vi "RIB Req - UDP Init.vi"(0 "Limits File Path":path, 5 "Results File Path":path, 11 "error in":errorcluster) -> (4 "Results Data Array":string[][](array[string]), 15 "error out":errorcluster)   [LabVIEW 2024]
doc: "Template test"
uses:
  <vilib>/addons/_JKI Toolkits/State Machine/_JKI_lib_State_Machine.llb/Select State(s)_err__jki_lib_state_machine.vi
  <vilib>/DAQmx/write.llb/DAQmx Write (Digital 1D Bool 1Chan 1Samp).vi
  <vilib>/addons/_JKI Toolkits/State Machine/_JKI_lib_State_Machine.llb/Select State(s)_bool__jki_lib_state_machine.vi
  <vilib>/DAQmx/read.llb/DAQmx Read (Digital 1D Bool 1Chan 1Samp).vi
  <vilib>/addons/_JKI Toolkits/State Machine/_JKI_lib_State_Machine.llb/Periodic Trigger__ogtk__JKI-SM__jki_lib_state_machine.vi
  <userlib>/_OpenG.lib/file/file.llb/Strip Path Extension - String__ogtk.vi
  <vilib>/Utility/file.llb/Read Delimited Spreadsheet (string).vi
  <vilib>/DAQmx/create/channels.llb/DAQmx Create Channel (DO-Digital Output).vi
  <vilib>/DAQmx/miscellaneous.llb/DAQmx Fill In Error Info.vi
  <userlib>/_OpenG.lib/file/file.llb/openg_file.lvlib
  <userlib>/_OpenG.lib/appcontrol/appcontrol.llb/openg_application_control.lvlib
  <userlib>/_OpenG.lib/time/time.llb/openg_time.lvlib
  <vilib>/Utility/file.llb/Write Delimited Spreadsheet (string).vi
panel:
  out "Connect Fail":string
  out "Connect":string
  out "Timeout (Read States) 4":dbl(slide) scale=0.0..30.0
  out "Timeout (Read States) 3":dbl(slide) scale=0.0..30.0
  out "Timeout (Read States) 2":dbl(slide) scale=0.0..30.0
  out "Timeout (Read States)":dbl(slide) scale=0.0..30.0
  out "element":string
  out "5A Test":bool
  out "ROV A Enabled":bool
  out "ROV B Enabled":bool
  out "TMS Enabled":bool
  out "Wait for Start":bool
  out "Normal Operation":bool
  in  "Read Normal Operation":string
  in  "Read Wait for Start":string
  in  "Read TMS":string
  in  "Read ROV B":string
  in  "Read ROV A":string
  in  "Connect":string
  in  "Connect Fail":string
  out "Results Data 10":string[](array[string])
  out "Results Data 9":string[](array[string])
  out "Results Data 8":string[](array[string])
  out "Results Data 7":string[](array[string])
  out "Results Data 6":string[](array[string])
  out "Results Data 5":string[](array[string])
  out "Results Data 4":string[](array[string])
  in  "5A Test":bool
  out "Results Data 3":string[](array[string])
  in  "task out":refnum<k21>
  out "Timeout (5A)":dbl(slide) scale=0.0..5.0
  out "Timeout (Read UDP)":dbl(slide) scale=0.0..20.0
  out "Results Data 2":string[](array[string])
  in  "UDP Read":string
  in  "connection ID":refnum<k16>
  in  "Exit":bool
  # "UDP Initialise Test"
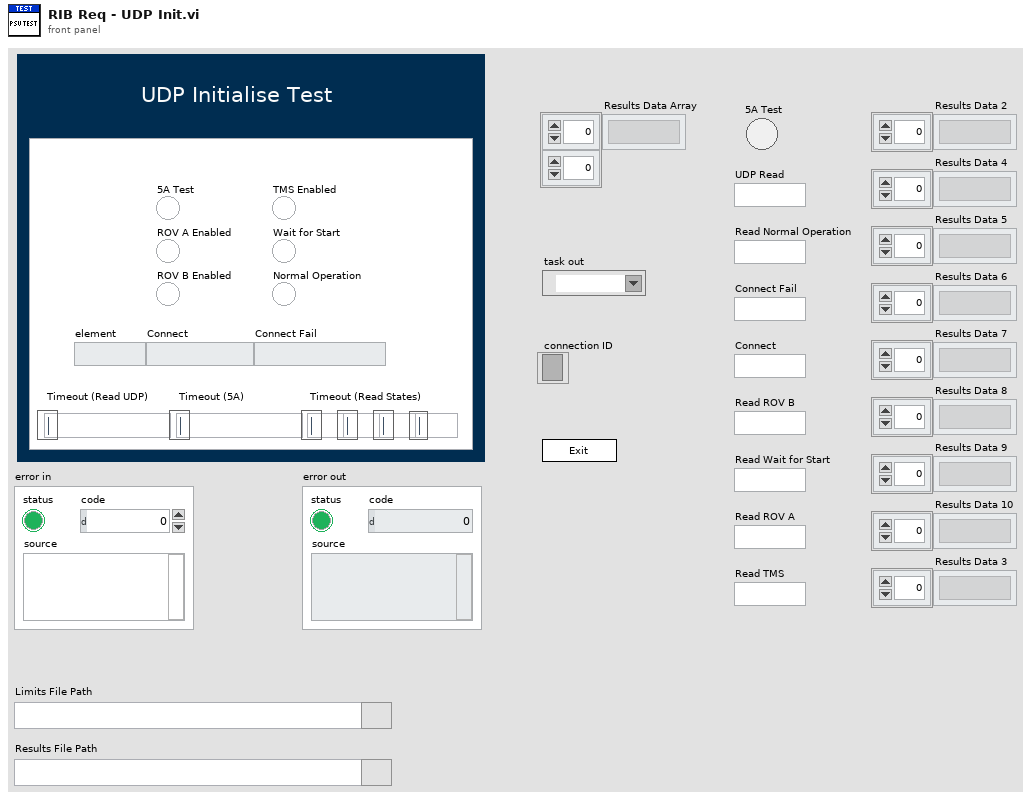
[diagram p1: front panel]
types:
  T1 = enum32{"Invalid", "Standard", "Closed", "Hidden", "Minimized", "Maximized"}
  T2 = enum32{"invalid app kind", "Development System", "Run Time System", "Student Edition", "Embedded LabVIEW", "Evaluation", "Custom"}
  T3 = typedef "FGV - Enum" = enum16{"Cleanup", "Get Data", "Open UDP", "Initialise DAQ", "Initialise I2C"}
  T4 = enum16{"Start Timer", "Get Time", "Pause", "Unpause"}
  T5 = cluster{"Core":cluster{"Current VI Reference":refnum<vi>, "Close Panel on Exit?":bool}, "Limits File Path":path, "Test Limits":string[][], "Results Data Array":string[][], "Results File Path":path, "UDP Read":string, "connection ID":refnum<k16>, "task out":refnum<k21>, "5A Test":bool, "Connect Fail":string, "Connect":string, "Read ROV A":string, "Read ROV B":string, "Read TMS":string, "Read Wait for Start":string, "Read Normal Operation":string}
  T6 = cluster{"Current VI Reference":refnum<vi>, "Close Panel on Exit?":bool}
  T7 = cluster{"[0]":bool, "[1]":bool, "[2]":bool, "[3]":bool, "[4]":bool, "[5]":bool, "[6]":bool, "[7]":bool, "[8]":bool}
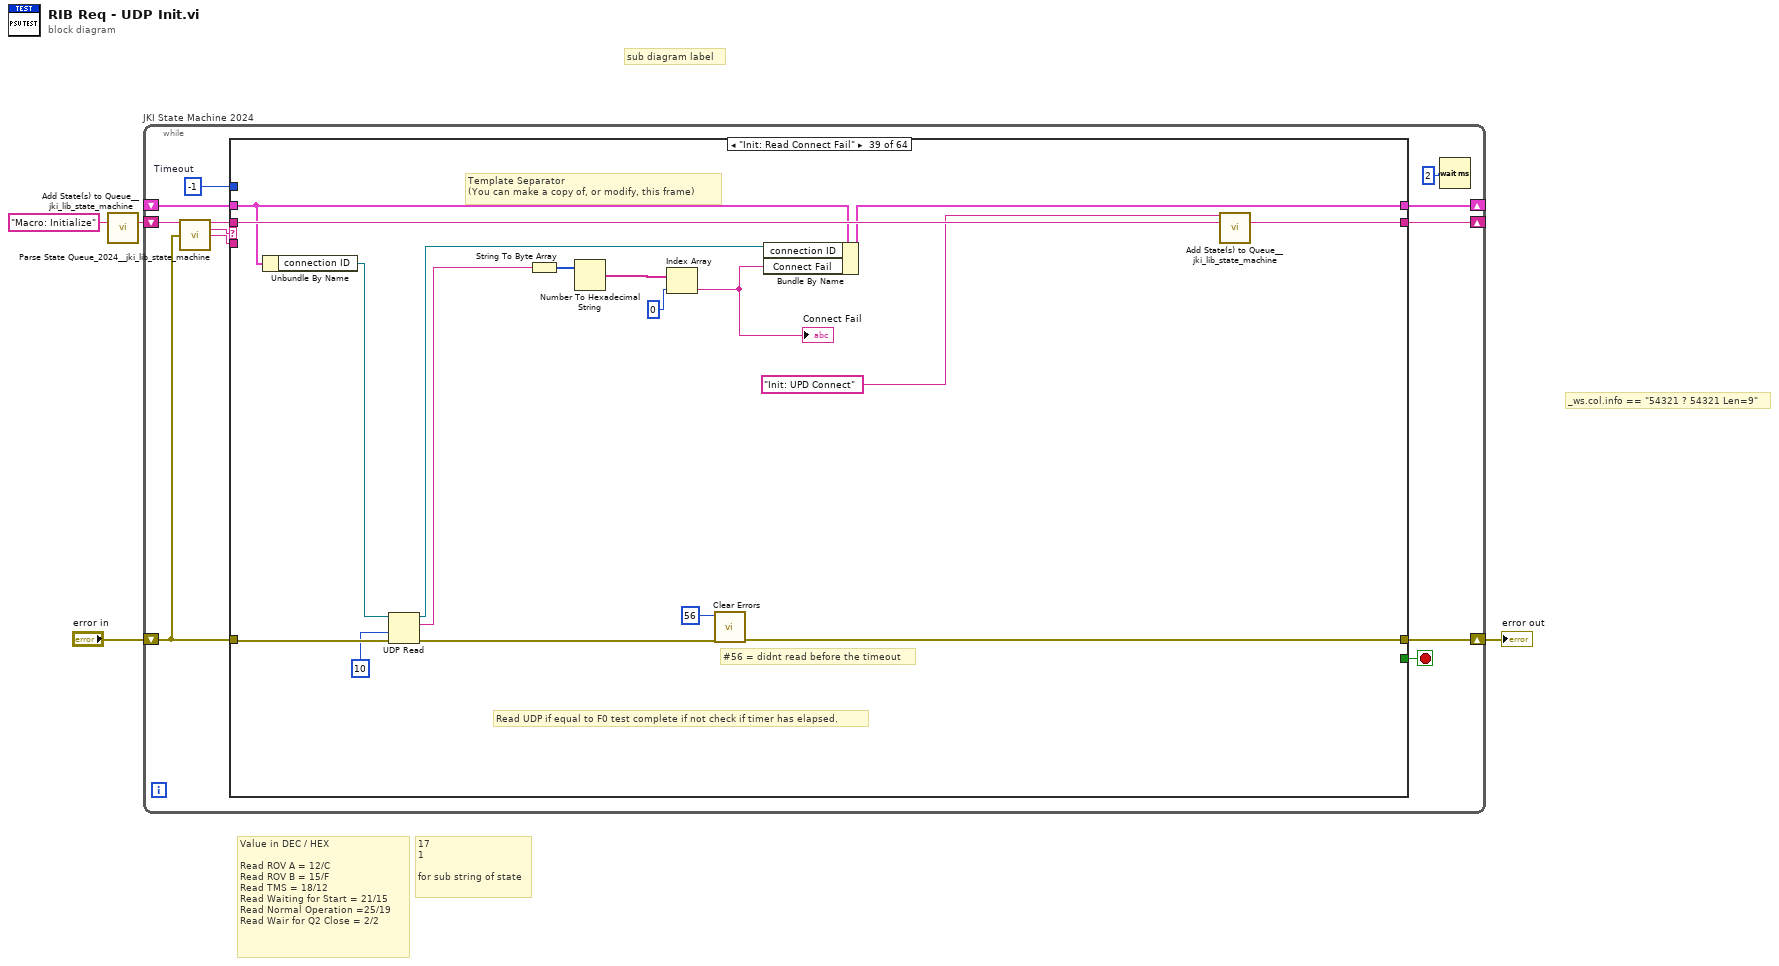
[diagram p0: block diagram]
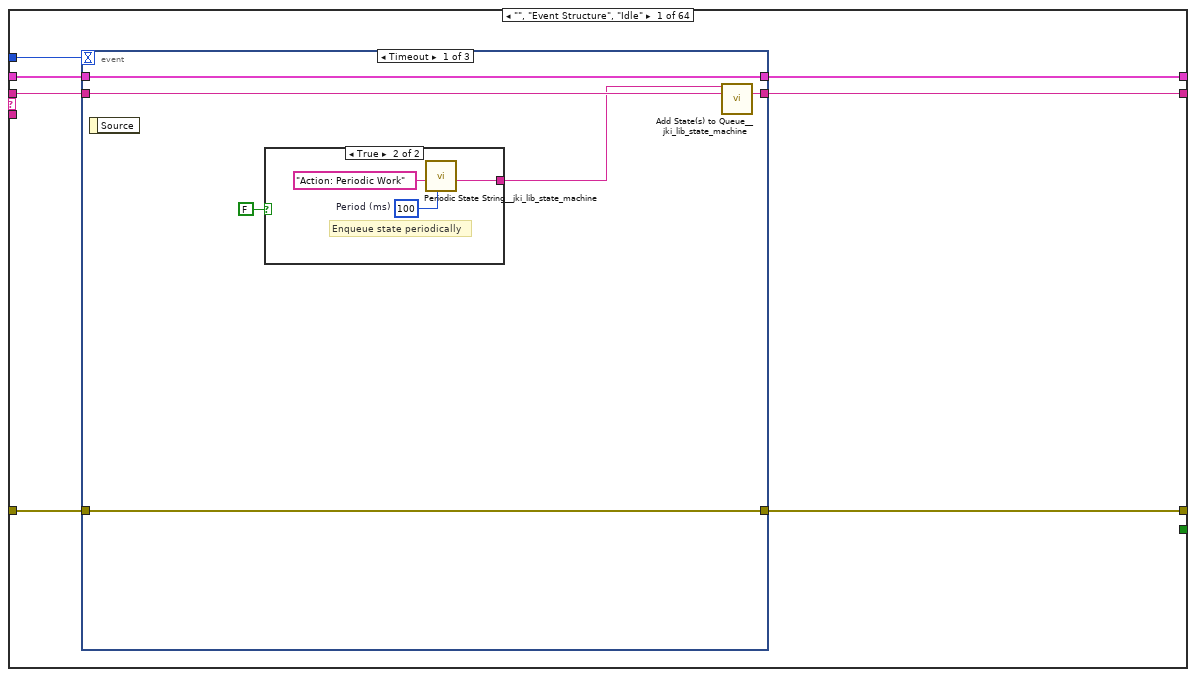
[diagram p2: hidden frame]
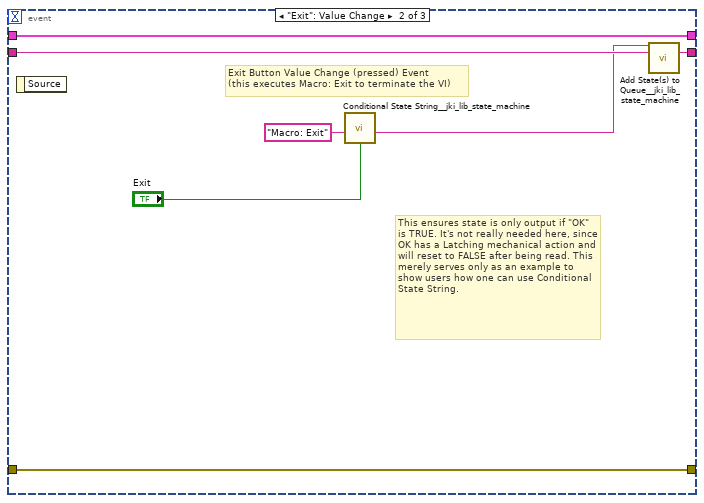
[diagram p4: hidden frame]
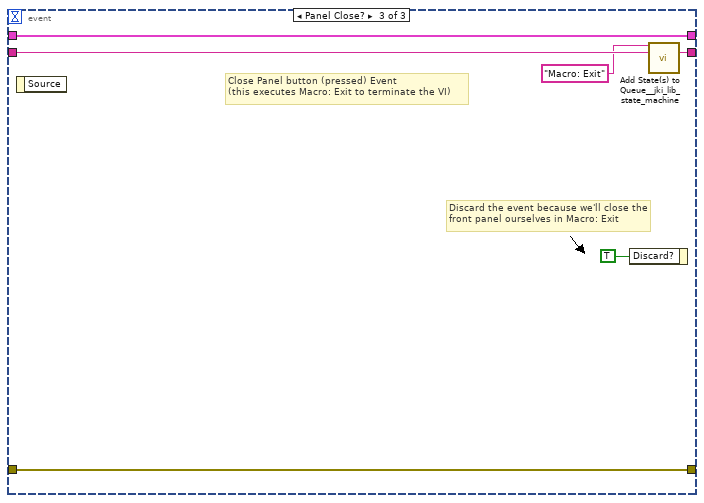
[diagram p5: hidden frame]
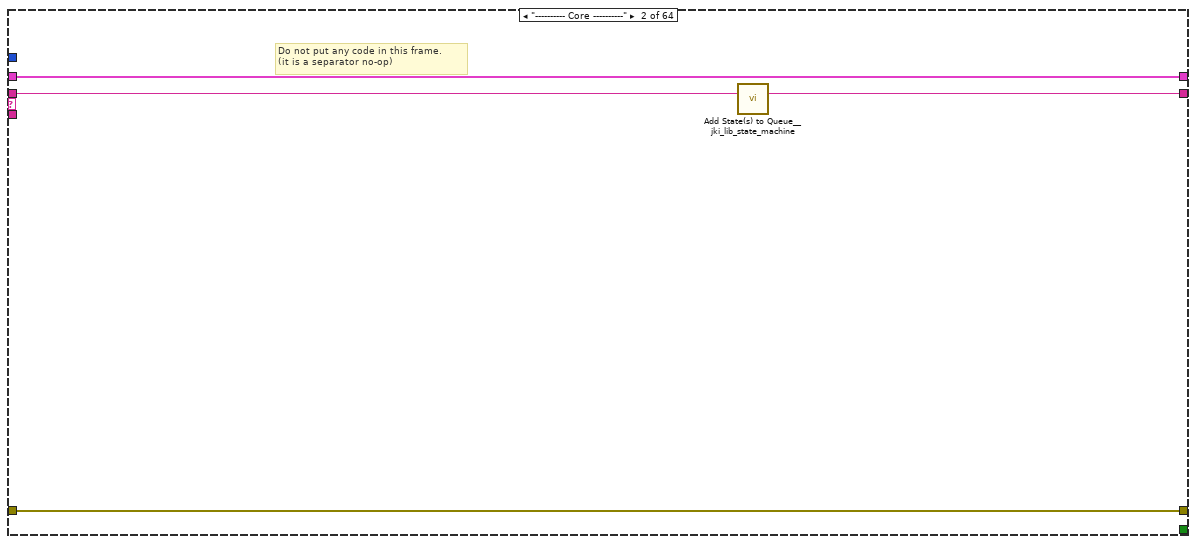
[diagram p6: hidden frame]
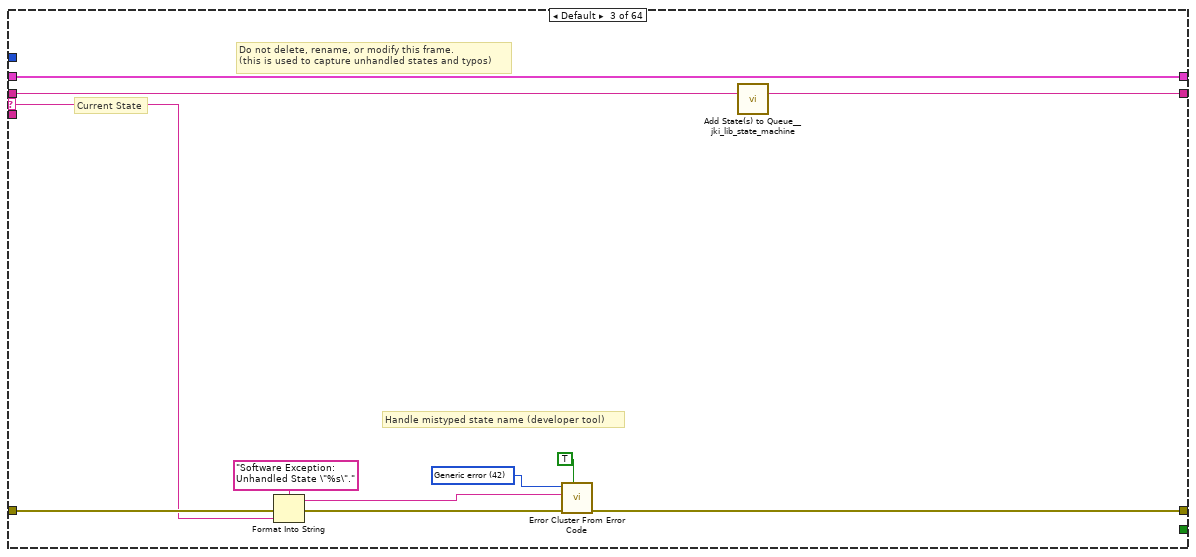
[diagram p7: hidden frame]
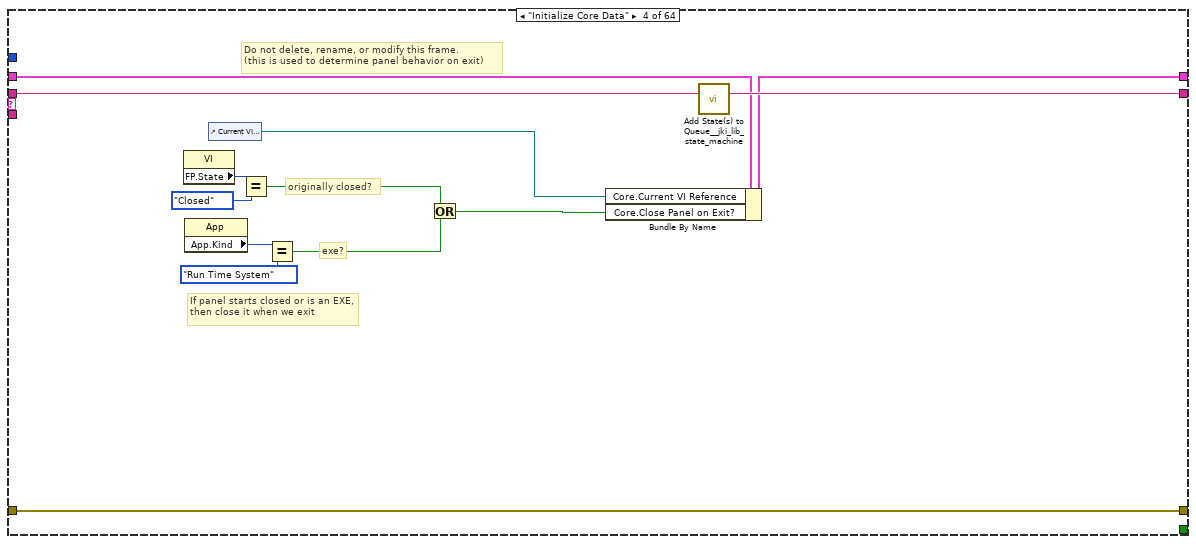
[diagram p8: hidden frame]
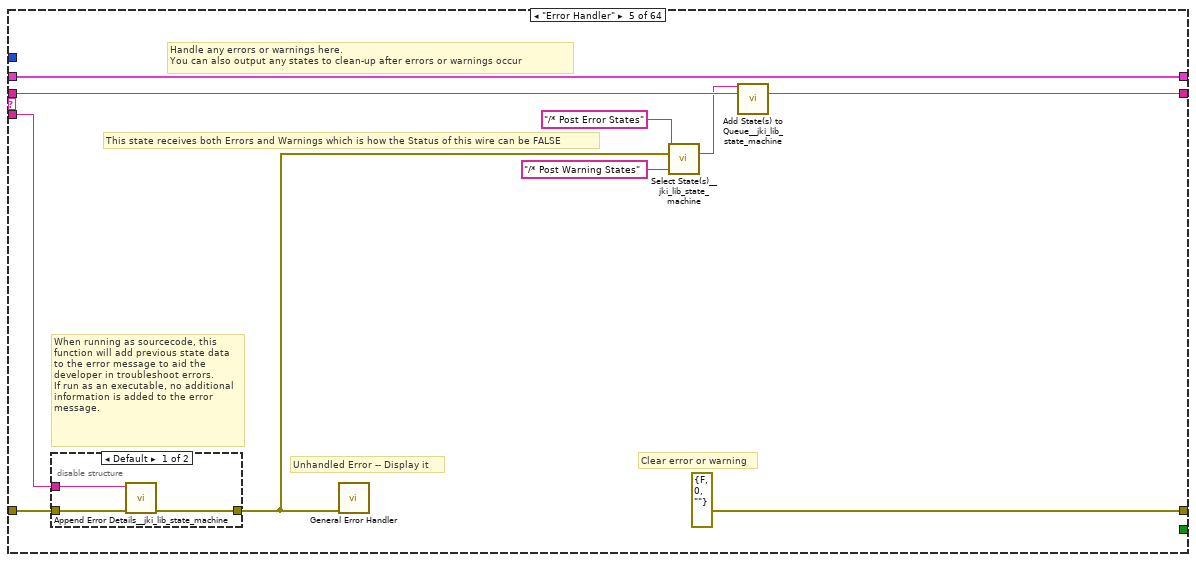
[diagram p9: hidden frame]
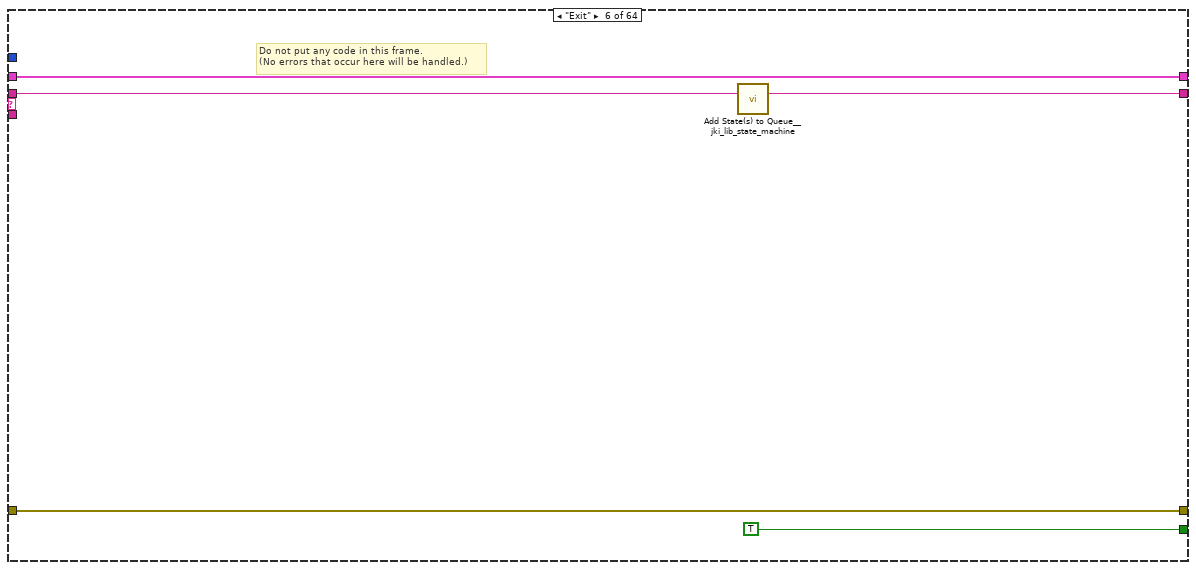
[diagram p11: hidden frame]
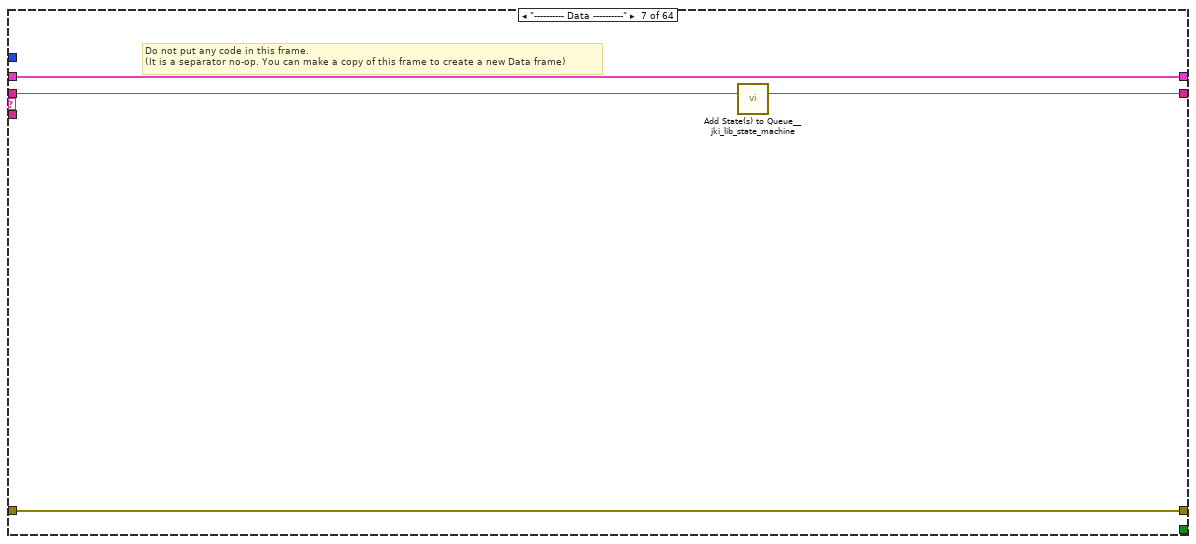
[diagram p12: hidden frame]
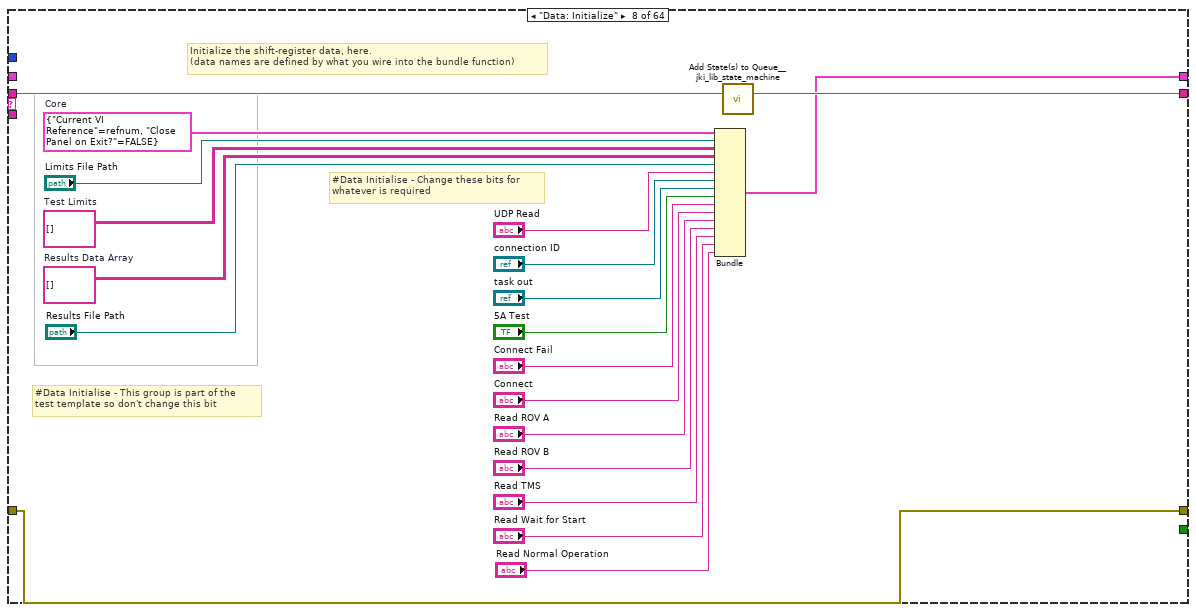
[diagram p13: hidden frame]
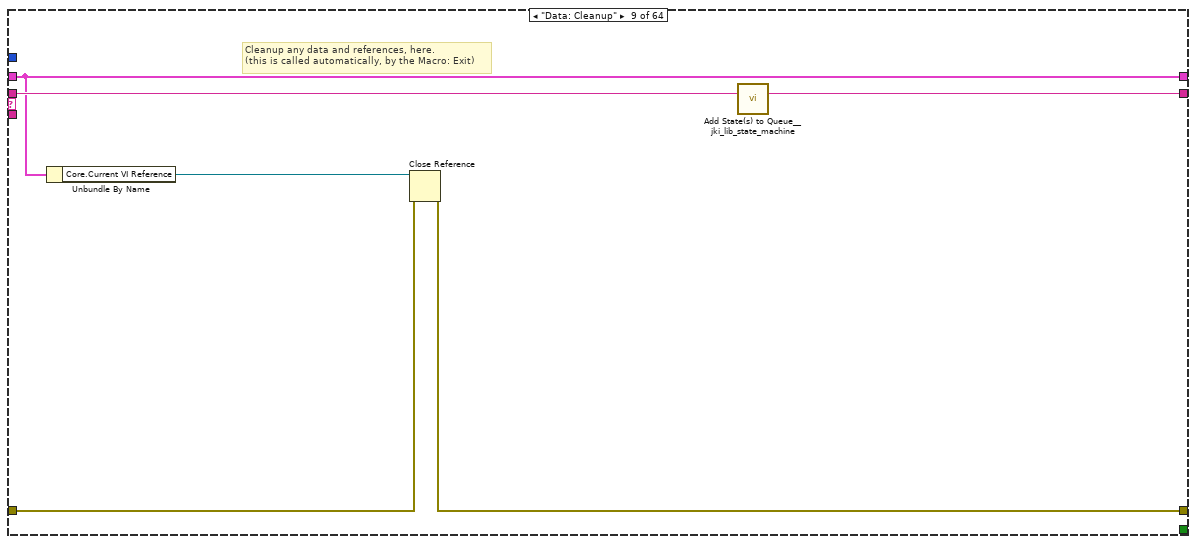
[diagram p14: hidden frame]
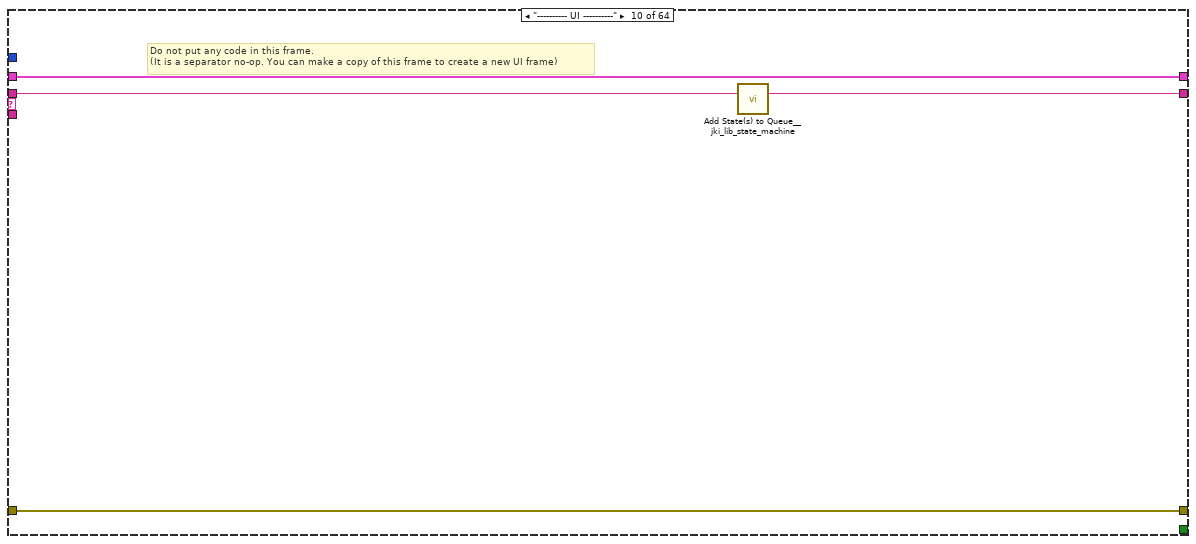
[diagram p15: hidden frame]
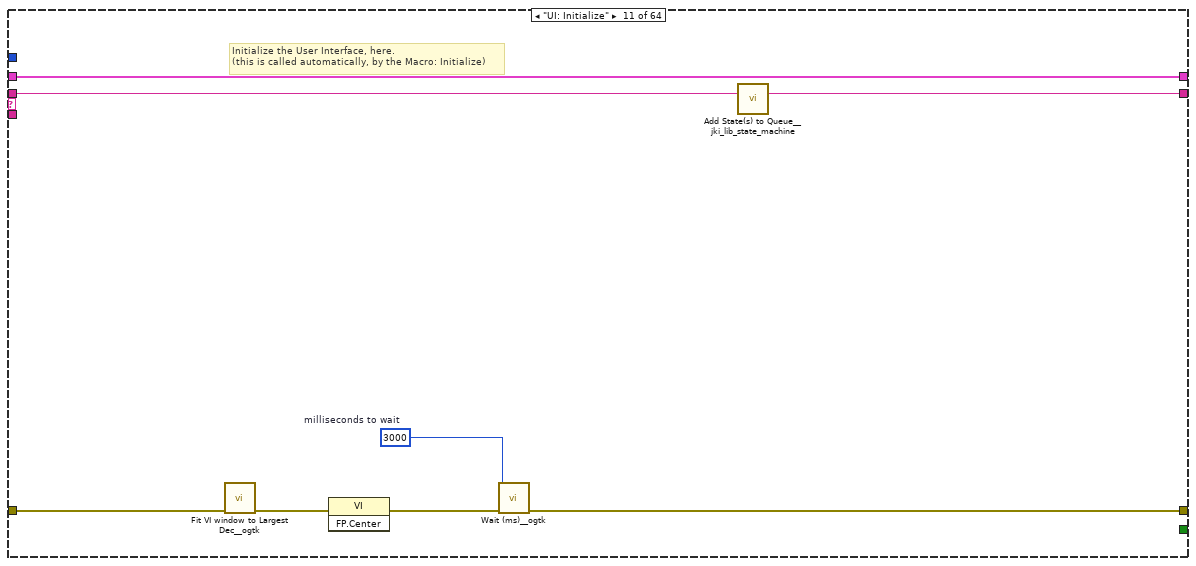
[diagram p16: hidden frame]
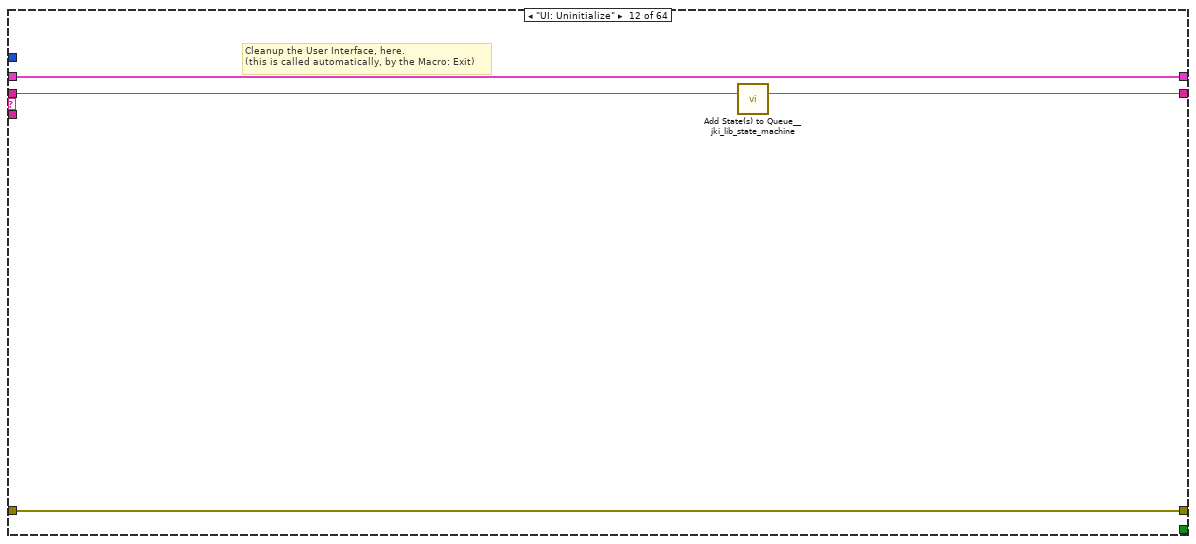
[diagram p17: hidden frame]
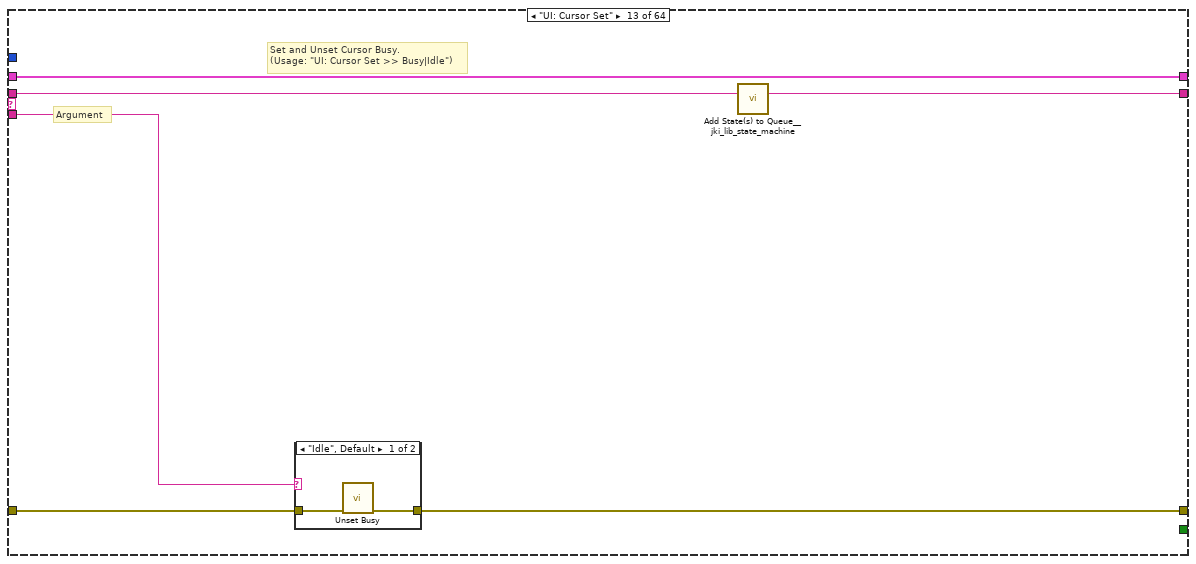
[diagram p18: hidden frame]
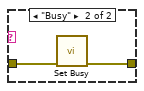
[diagram p19: hidden frame]
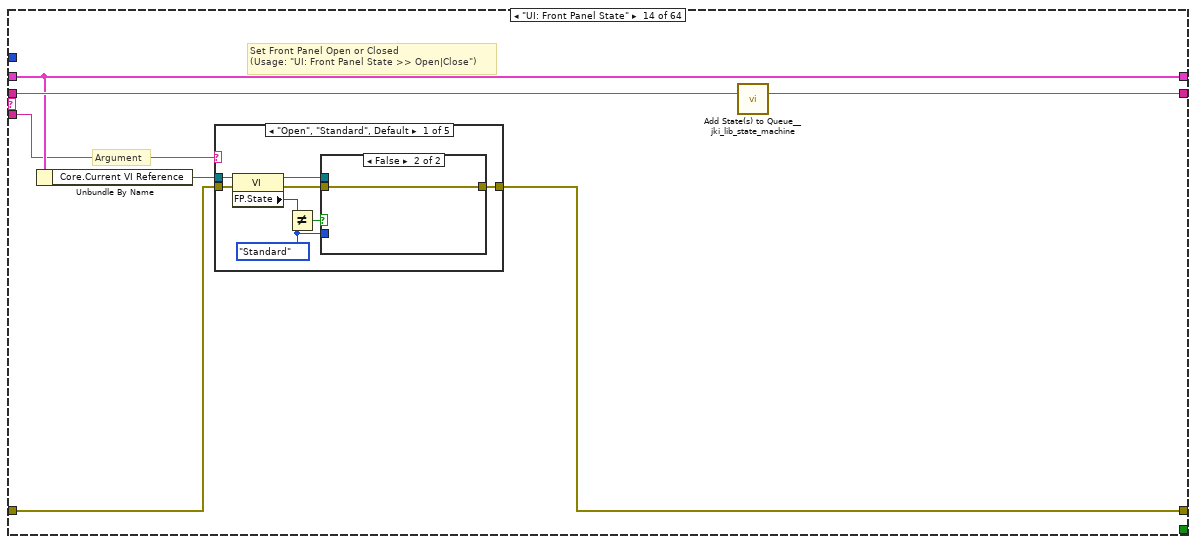
[diagram p20: hidden frame]
diagram:
  # "17\n1\n\nfor sub string of state"
  # "Value in DEC / HEX\n\nRead ROV A = 12/C\nRead ROV B = 15/F\nRead TMS = 18/12\nRead Waiting for Start = 21/15\nRead Normal Operation =25/19 \nRead Wair for Q2 Close = 2/2"
  # "_ws.col.info == \"54321 ? 54321 Len=9\""
  # "sub diagram label"
  n1 = call <vilib>:"Add State(s) to Queue__jki_lib_state_machine.vi"("State(s) in (\"\")"="Macro: Initialize") -> ("States Out"=w4:string)  [unwired: 14 in]
  n2 = while "JKI State Machine 2024" {
    shift-right: [w9] -> _
    shift-left: _ -> [w8]
    shift-right: [w12] -> w1
    shift-left: "error in" -> [w6]
    shift-right: [w11] -> _
    shift-left: w4 -> [w13]
    stop <- w10 stop-if-true
    w7 = -1  # Timeout
    n3 = call <vilib>:"Parse State Queue_2024__jki_lib_state_machine.vi"("State Queue"=w13, "Error In (no error)"=w6) -> ("Remaining States"=w15:string, "Current State"=w16:string, "Arguments"=w14:string)  [unwired: 11 in]
    n4 = case shown="\"Init: Read Connect Fail\"" w16 {
      selector: w16 -> [_ _ w50 _ _ _ _ _ _ _ _ _ _ _ _ _ _ _ _ _ _ _ _ _ _ _ _ _ _ _ _ _ _ _ _ _ _ _ _ _ _ _ _ _ _ _ _ _ _ _ _ _ _ _ _ _ _ _ _ _ _ _ _ _]
      tunnel: w15 -> [w23 w49 w54 w73 w83 w92 w96 w116 w122 w126 w134 w138 w144 w155 w224 w229 w234 w239 w248 w252 w265 w282 w295 w308 w321 w334 w347 w360 w373 w386 w390 w399 w403 w419 w426 w439 w448 w472 w489 w513 w530 w541 w562 w586 w598 w609 w629 w641 w686 w708 w719 w743 w755 w766 w790 w802 w813 w837 w849 w860 w884 w896 w918 w940]
      tunnel: w14 -> [_ _ _ _ w78 _ _ _ _ _ _ _ w139 w149 _ _ _ _ _ _ _ _ _ _ _ _ _ _ _ _ _ _ _ _ _ _ _ _ _ _ _ _ _ _ _ _ _ _ _ _ _ _ _ _ _ _ _ _ _ _ _ _ _ _]
      tunnel: w8 -> [w21 w46 w52 w66 w80 w90 w93 _ w117 w123 w132 w136 w142 w151 w221 w226 w231 w236 w246 w249 w255 w274 w287 w300 w313 w326 w339 w352 w365 w378 w387 w395 w400 w417 w422 w434 w446 w453 w485 w494 w526 w539 w545 w580 w596 w607 w625 w639 w650 w705 w717 w729 w753 w764 w773 w800 w811 w820 w847 w858 w867 w894 w915 w927]
      tunnel: [w20 w47 w56 w70 errorcluster {"status"=FALSE, "code"=0, "source"=""} ("error out") w89 w94 w113 w118 w124 w130 w135 w140 w152 w222 w227 w232 w237 w243 w250 w261 w279 w292 w305 w318 w331 w344 w357 w370 w383 w388 w397 w401 w407 w421 w430 w443 w449 w478 w490 w522 w532 w542 w566 w593 w599 w614 w636 w644 w688 w710 w727 w750 w757 w769 w797 w804 w816 w844 w851 w863 w891 w898 w922] -> w12
      tunnel: w6 -> [w17 w47 w55 w70 w79 w89 w94 w113 w119 w124 w131 w135 w141 w153 w222 w227 w232 w237 w243 w250 w260 w278 w291 w304 w317 w330 w343 w356 w369 w382 w388 w396 w401 w412 w421 w435 w442 w454 w487 w495 w528 w537 w547 w582 w594 w605 w615 w637 w653 w694 w715 w726 w751 w762 w768 w798 w809 w815 w845 w856 w862 w892 w904 w924]
      tunnel: [w22 w48 w53 w72 w82 w91 w95 w115 w121 w125 w133 w137 w143 w154 w223 w228 w233 w238 w247 w251 w264 w281 w294 w307 w320 w333 w346 w359 w372 w385 w389 w398 w402 w418 w425 w438 w447 w471 w488 w512 w529 w540 w561 w585 w597 w608 w628 w640 w685 w707 w718 w742 w754 w765 w789 w801 w812 w836 w848 w859 w883 w895 w917 w939] -> w11
      tunnel: [_ _ _ _ _ TRUE _ _ _ _ _ _ _ _ _ _ _ _ _ _ _ _ _ _ _ _ _ _ _ _ _ _ _ _ _ _ _ _ _ _ _ _ _ _ _ _ _ _ _ _ _ _ _ _ _ _ _ _ _ _ _ _ _ _] -> w10
      tunnel: [w19 w46 w52 w71 w80 w90 w93 w114 w117 w123 w132 w136 w142 w151 w221 w226 w231 w236 w246 w249 w254 w273 w286 w299 w312 w325 w338 w351 w364 w377 w387 w395 w400 w417 w422 w433 w445 w455 w484 w496 w525 w539 w549 w579 w596 w607 w624 w639 w684 w706 w717 w728 w753 w764 w772 w800 w811 w819 w847 w858 w866 w894 w916 w926] -> w9
      tunnel: w7 -> [w18 _ _ _ _ _ _ _ _ _ _ _ _ _ _ _ _ _ _ _ _ _ _ _ _ _ _ _ _ _ _ _ _ _ _ _ _ _ _ _ _ _ _ _ _ _ _ _ _ _ _ _ _ _ _ _ _ _ _ _ _ _ _ _]
      frame "", "Event Structure", "Idle" {
        n5 = event shown="[0] Timeout" {
          selector: _ -> [_ _ _]
          dyn-events: _ -> [_ _ _]
          timeout: w18 -> [_ _ _]
          tunnel: w23 -> [w29 w39 w45]
          tunnel: [w28 w38 w44] -> w22
          tunnel: w21 -> [w26 w36 w42]
          tunnel: [w27 w37 w43] -> w20
          tunnel: w17 -> [w27 w37 w43]
          tunnel: [w26 w36 w42] -> w19
          event Timeout {
            n6 = event-data() -> ()  [unwired: 1 in, 1 out]
            n7 = case shown="True" FALSE {
              tunnel: [_ w32] -> w25
              frame False {
              }
              frame True {
                w30 = u32 100  # Period (ms)
                # "Enqueue state periodically"
                n8 = call <vilib>:"Periodic State String__jki_lib_state_machine.vi"("Period (ms)"=w30, "State"="Action: Periodic Work") -> ("State Out"=w32:string)  [unwired: 9 in]
              }
            }
            n9 = call <vilib>:"Add State(s) to Queue__jki_lib_state_machine.vi"("State(s) in Front (\"\")"=w25, "State(s) in (\"\")"=w29) -> ("States Out"=w28:string)  [unwired: 13 in]
          }
          event "Exit": Value Change {
            # "This ensures state is only output if \"OK\" is TRUE. It's not really needed here, since OK has a Latching mechanical action and will reset to FALSE after being read. This merely serves only as an example to show users how one can use Conditional State String."
            # "Exit Button Value Change (pressed) Event\n(this executes Macro: Exit to terminate the VI)"
            n10 = event-data() -> ()  [unwired: 1 in, 1 out]
            n11 = call <vilib>:"Conditional State String__jki_lib_state_machine.vi"("Do State(s)?"="Exit", "State"="Macro: Exit") -> ("State Out"=w33:string)  [unwired: 7 in]
            n12 = call <vilib>:"Add State(s) to Queue__jki_lib_state_machine.vi"("State(s) in Front (\"\")"=w33, "State(s) in (\"\")"=w39) -> ("States Out"=w38:string)  [unwired: 13 in]
          }
          event Panel Close? {
            # "Discard the event because we'll close the front panel ourselves in Macro: Exit"
            # "Close Panel button (pressed) Event\n(this executes Macro: Exit to terminate the VI)"
            n13 = event-data() -> ()  [unwired: 1 in, 1 out]
            n14 = event-data("Discard?"=TRUE) -> ()  [unwired: 1 in, 1 out]
            n15 = call <vilib>:"Add State(s) to Queue__jki_lib_state_machine.vi"("State(s) in Front (\"\")"="Macro: Exit", "State(s) in (\"\")"=w45) -> ("States Out"=w44:string)  [unwired: 13 in]
          }
        }
      }
      frame "---------- Core ----------" {
        # "Do not put any code in this frame.\n(it is a separator no-op)"
        n16 = call <vilib>:"Add State(s) to Queue__jki_lib_state_machine.vi"("State(s) in (\"\")"=w49) -> ("States Out"=w48:string)  [unwired: 14 in]
      }
      frame Default {
        w59 = 42 items=["No error", "Argument error", "Memory is full", "Out of zone", "End of file", "File already open", "Generic file I/O error", "File not found", "File permission error", "Disk is full", "Duplicate path", "Too many files open", "System feature not enabled", "Resource file not found", "Cannot add resource", "Resource not found", "Image not found", "Image memory error", "Pen does not exist", "Config type invalid", "Config token not found", "Config parse error", "Config memory error", "Bad external code format", "Bad external code offset", "External code not present", "Null window", "Destroy window error", "Null menu", "Print aborted", "Bad print record", "Print driver error", "Windows error during printing", "Memory error during printing", "Print dialog error", "Generic print error", "Invalid device refnum", "Device not found", "Device parameter error", "Device unit error", "Cannot open device", "Device call aborted", "Generic error", "Cancelled by user", "Object ID too low", "Object ID too high", "Object not in heap", "Unknown heap", "Unknown object (invalid DefProc)", "Unknown object (DefProc not in table)", "Message out of range", "Invalid (null) method", "Unknown message", "Manager call not supported", "Bad address", "Network operation in progress", "Network operation timed out", "Connection is busy", "Network attribute not supported", "Network error", "Address in use", "System out of memory", "Connection aborted", "Connection refused", "Not connected", "Already connected", "Connection closed", "Initialization error (interapplication manager)", "Bad occurrence", "Wait on unbound occurrence handler", "Occurrence queue overflow", "Datalog type conflict", "Unused", "Unrecognized type (interapplication manager)", "Memory corrupt", "Failed to make temporary DLL", "Old CIN version", "Drag socket not found", "Failed to load drop-object", "Failed to register OLE object", "Failed to release OLE object", "Format specifier type mismatch", "Unknown format specifier", "Too few format specifiers", "Too many format specifiers", "Scan failed", "Newer CIN version", "Error converting to variant", "Runtime menu error", "Password tampered", "Variant attribute not found", "Incompatible variant data type", "Event data is not available", "Event Store is not present", "Occurrence is not found", "Event Queue is not created", "Event info is not available", "Refnum passed is NULL", "Error retrieving Class GUID", "Error retrieving CoClass GUID", "Error retrieving TypeLib GUID.", "Bad built application magic bytes.", "Specific driver is different from the specific driver associated with the Logical Name.", "There is no session opened to the class driver.", "Max Error", "MAX - Error with config objects", "MAX - Error loading configuration", "MAX - Group not supported"]
        # "Current State"
        # "Do not delete, rename, or modify this frame.\n(this is used to capture unhandled states and typos)"
        # "Handle mistyped state name (developer tool)"
        n17 = Format Into String(format string="Software Exception: Unhandled State \"%s\"." ("message"), error in=w55, w50) -> (resulting string=w58:string, error out=w57:errorcluster)  [unwired: 1 in]
        n18 = call <vilib>:"Error Cluster From Error Code.vi"("show call chain? (False)"=TRUE, "error in (no error)"=w57, "error message (\"\")"=w58, "error code (0)"=w59) -> ("error out"=w56:errorcluster)  [unwired: 5 in]
        n19 = call <vilib>:"Add State(s) to Queue__jki_lib_state_machine.vi"("State(s) in (\"\")"=w54) -> ("States Out"=w53:string)  [unwired: 14 in]
      }
      frame "Initialize Core Data" {
        # "Do not delete, rename, or modify this frame.\n(this is used to determine panel behavior on exit)"
        # "originally closed?"
        # "exe?"
        # "If panel starts closed or is an EXE, then close it when we exit"
        n20 = property class="VI"() -> ("FP.State"=w63:T1)  [unwired: 2 in, 2 out]
        n21 = property class="App"() -> ("App.Kind"=w69:T2)  [unwired: 2 in, 2 out]
        n22 = control-ref of="Current VI Reference"() -> (w64:refnum<vi>)
        n23 = Equal?(x=w63, y=T1."Closed" ("Front Panel Window:State")) -> (x = y?=w61:bool)
        n24 = Equal?(x=w69, y=T2."Run Time System" ("Application:Kind")) -> (x = y?=w67:bool)
        n25 = Or(x=w61, y=w67) -> (x .or. y?=w65:bool)
        n26 = Bundle By Name(cluster=w66, "Core.Current VI Reference"=w64, "Core.Close Panel on Exit?"=w65) -> (w71:T5)
        n27 = call <vilib>:"Add State(s) to Queue__jki_lib_state_machine.vi"("State(s) in (\"\")"=w73) -> ("States Out"=w72:string)  [unwired: 14 in]
      }
      frame "Error Handler" {
        # "When running as sourcecode, this function will add previous state data to the error message to aid the developer in troubleshoot errors.\nIf run as an executable, no additional information is added to the error message."
        # "This state receives both Errors and Warnings which is how the Status of this wire can be FALSE"
        # "Unhandled Error -- Display it"
        # "Handle any errors or warnings here.\nYou can also output any states to clean-up after errors or warnings occur"
        # "Clear error or warning"
        n28 = disable-structure shown="Default" {
          disable-tunnel: w79 -> [w86 w87]
          disable-tunnel: w78 -> [w85 _]
          disable-tunnel: [w84 w87] -> w77
          frame condition #0 (active) {
            n29 = call <vilib>:"Append Error Details__jki_lib_state_machine.vi"("error in (no error)"=w86, "Previous State and Argument(s)"=w85) -> ("error out"=w84:errorcluster)  [unwired: 9 in]
          }
          frame condition #1 {
          }
        }
        n30 = call <vilib>:"General Error Handler.vi"("error in (no error)"=w77) -> ()  [unwired: 10 in, 5 out]
        n31 = call-poly <vilib>:"Select State(s)__jki_lib_state_machine.vi"("State(s) if True (\"\")"="/* Post Error States", "Select"=w77, "State(s) if False (\"\")"="/* Post Warning States") -> ("States Out"=w75:string)  [unwired: 12 in]
        n32 = call <vilib>:"Add State(s) to Queue__jki_lib_state_machine.vi"("State(s) in Front (\"\")"=w75, "State(s) in (\"\")"=w83) -> ("States Out"=w82:string)  [unwired: 13 in]
      }
      frame "Exit" {
        # "Do not put any code in this frame.\n(No errors that occur here will be handled.)"
        n33 = call <vilib>:"Add State(s) to Queue__jki_lib_state_machine.vi"("State(s) in (\"\")"=w92) -> ("States Out"=w91:string)  [unwired: 14 in]
      }
      frame "---------- Data ----------" {
        # "Do not put any code in this frame.\n(It is a separator no-op. You can make a copy of this frame to create a new Data frame)"
        n34 = call <vilib>:"Add State(s) to Queue__jki_lib_state_machine.vi"("State(s) in (\"\")"=w96) -> ("States Out"=w95:string)  [unwired: 14 in]
      }
      frame "Data: Initialize" {
        w109 = string[][] []  # Results Data Array
        w110 = string[][] []  # Test Limits
        w112 = T6 {"Current VI Reference"=refnum, "Close Panel on Exit?"=FALSE}  # Core
        # "#Data Initialise - Change these bits for\nwhatever is required"
        # "#Data Initialise - This group is part of the\ntest template so don't change this bit"
        # "Initialize the shift-register data, here.\n(data names are defined by what you wire into the bundle function)"
        n35 = Bundle("Core"=w112, "Limits File Path"="Limits File Path", "Test Limits"=w110, "Results Data Array"=w109, "Results File Path"="Results File Path", "UDP Read"="UDP Read", "connection ID"="connection ID", "task out"="task out", "5A Test"="5A Test", "Connect Fail"="Connect Fail", "Connect"="Connect", "Read ROV A"="Read ROV A", "Read ROV B"="Read ROV B", "Read TMS"="Read TMS", "Read Wait for Start"="Read Wait for Start", "Read Normal Operation"="Read Normal Operation") -> (w114:T5)  [unwired: 1 in]
        n36 = call <vilib>:"Add State(s) to Queue__jki_lib_state_machine.vi"("State(s) in (\"\")"=w116) -> ("States Out"=w115:string)  [unwired: 14 in]
      }
      frame "Data: Cleanup" {
        # "Cleanup any data and references, here.\n(this is called automatically, by the Macro: Exit)"
        n37 = Unbundle By Name(w117) -> ("Core.Current VI Reference"=w120:refnum<vi>)
        n38 = Close Reference(reference=w120, error in (no error)=w119) -> (error out=w118:errorcluster)
        n39 = call <vilib>:"Add State(s) to Queue__jki_lib_state_machine.vi"("State(s) in (\"\")"=w122) -> ("States Out"=w121:string)  [unwired: 14 in]
      }
      frame "---------- UI ----------" {
        # "Do not put any code in this frame.\n(It is a separator no-op. You can make a copy of this frame to create a new UI frame)"
        n40 = call <vilib>:"Add State(s) to Queue__jki_lib_state_machine.vi"("State(s) in (\"\")"=w126) -> ("States Out"=w125:string)  [unwired: 14 in]
      }
      frame "UI: Initialize" {
        w129 = u32 3000  # milliseconds to wait
        # "Initialize the User Interface, here.\n(this is called automatically, by the Macro: Initialize)"
        n41 = call <userlib>:"Fit VI window to Largest Dec__ogtk.vi"("error in (no error)"=w131) -> ("error out"=w127:errorcluster)  [unwired: 5 in, 1 out]
        n42 = invoke class="VI" method="FP.Center"(error in=w127) -> (error out=w128:errorcluster)  [unwired: 2 in, 2 out]
        n43 = call <userlib>:"Wait (ms)__ogtk.vi"("error in (no error)"=w128, "milliseconds to wait"=w129) -> ("error out"=w130:errorcluster)  [unwired: 8 in, 1 out]
        n44 = call <vilib>:"Add State(s) to Queue__jki_lib_state_machine.vi"("State(s) in (\"\")"=w134) -> ("States Out"=w133:string)  [unwired: 14 in]
      }
      frame "UI: Uninitialize" {
        # "Cleanup the User Interface, here.\n(this is called automatically, by the Macro: Exit)"
        n45 = call <vilib>:"Add State(s) to Queue__jki_lib_state_machine.vi"("State(s) in (\"\")"=w138) -> ("States Out"=w137:string)  [unwired: 14 in]
      }
      frame "UI: Cursor Set" {
        # "Argument"
        # "Set and Unset Cursor Busy.\n(Usage: \"UI: Cursor Set >> Busy|Idle\")"
        n46 = case shown="\"Idle\", Default" w139 {
          tunnel: w141 -> [w146 w148]
          tunnel: [w145 w147] -> w140
          frame "Idle", Default {
            n47 = call <vilib>:"Unset Busy.vi"("error in (no error)"=w146) -> ("error out"=w145:errorcluster)  [unwired: 10 in]
          }
          frame "Busy" {
            n48 = call <vilib>:"Set Busy.vi"("error in (no error)"=w148) -> ("error out"=w147:errorcluster)  [unwired: 9 in, 1 out]
          }
        }
        n49 = call <vilib>:"Add State(s) to Queue__jki_lib_state_machine.vi"("State(s) in (\"\")"=w144) -> ("States Out"=w143:string)  [unwired: 14 in]
      }
      frame "UI: Front Panel State" {
        # "Argument"
        # "Set Front Panel Open or Closed\n(Usage: \"UI: Front Panel State >> Open|Close\")"
        n50 = Unbundle By Name(w151) -> ("Core.Current VI Reference"=w150:refnum<vi>)
        n51 = case shown="\"Open\", \"Standard\", Default" w149 {
          tunnel: w153 -> [w161 w176 w187 w200 w213]
          tunnel: [w163 w177 w189 w202 w215] -> w152
          tunnel: w150 -> [w162 w174 w188 w201 w214]
          frame "Open", "Standard", Default {
            w156 = T1."Standard" ("State")
            n52 = property class="VI"(reference=w162, error in=w161) -> (reference out=w159:refnum<vi>, error out=w160:errorcluster, "FP.State"=w158:T1)
            n53 = Not Equal?(x=w158, y=w156) -> (x != y?=w157:bool)
            n54 = case shown="False" w157 {
              tunnel: [w167 w169] -> w163
              tunnel: w160 -> [w166 w169]
              tunnel: w159 -> [w165 _]
              tunnel: w156 -> [w164 _]
              frame True {
                n55 = invoke class="VI" method="FP.Open"(reference=w165, error in=w166, "Activate"=TRUE, "State"=w164) -> (error out=w167:errorcluster)  [unwired: 1 in, 4 out]
              }
              frame False {
              }
            }
          }
          frame "Close", "Closed" {
            n56 = property class="VI"(reference=w174, error in=w176) -> (reference out=w173:refnum<vi>, error out=w175:errorcluster, "FP.State"=w171:T1)
            n57 = Not Equal?(x=w171, y=T1."Closed" ("Front Panel Window:State")) -> (x != y?=w170:bool)
            n58 = case shown="True" w170 {
              tunnel: [w178 w181] -> w177
              tunnel: w175 -> [w178 w180]
              tunnel: w173 -> [_ w179]
              frame False {
              }
              frame True {
                n59 = invoke class="VI" method="FP.Close"(reference=w179, error in=w180) -> (error out=w181:errorcluster)  [unwired: 1 in, 2 out]
              }
            }
          }
          frame "Hidden", "Hide" {
            w182 = T1."Hidden" ("State")
            n60 = property class="VI"(reference=w188, error in=w187) -> (reference out=w185:refnum<vi>, error out=w186:errorcluster, "FP.State"=w184:T1)
            n61 = Not Equal?(x=w184, y=w182) -> (x != y?=w183:bool)
            n62 = case shown="True" w183 {
              tunnel: [w193 w194] -> w189
              tunnel: w186 -> [w192 w194]
              tunnel: w185 -> [w191 _]
              tunnel: w182 -> [w190 _]
              frame True {
                n63 = invoke class="VI" method="FP.Open"(reference=w191, error in=w192, "State"=w190) -> (error out=w193:errorcluster)  [unwired: 2 in, 4 out]
              }
              frame False {
              }
            }
          }
          frame "Minimize", "Minimized" {
            w195 = T1."Minimized" ("State")
            n64 = property class="VI"(reference=w201, error in=w200) -> (reference out=w198:refnum<vi>, error out=w199:errorcluster, "FP.State"=w197:T1)
            n65 = Not Equal?(x=w197, y=w195) -> (x != y?=w196:bool)
            n66 = case shown="True" w196 {
              tunnel: [w206 w207] -> w202
              tunnel: w199 -> [w205 w207]
              tunnel: w198 -> [w204 _]
              tunnel: w195 -> [w203 _]
              frame True {
                n67 = invoke class="VI" method="FP.Open"(reference=w204, error in=w205, "State"=w203) -> (error out=w206:errorcluster)  [unwired: 2 in, 4 out]
              }
              frame False {
              }
            }
          }
          frame "Maximize", "Maximized" {
            w208 = T1."Maximized" ("State")
            n68 = property class="VI"(reference=w214, error in=w213) -> (reference out=w211:refnum<vi>, error out=w212:errorcluster, "FP.State"=w210:T1)
            n69 = Not Equal?(x=w210, y=w208) -> (x != y?=w209:bool)
            n70 = case shown="True" w209 {
              tunnel: [w219 w220] -> w215
              tunnel: w212 -> [w218 w220]
              tunnel: w211 -> [w217 _]
              tunnel: w208 -> [w216 _]
              frame True {
                n71 = invoke class="VI" method="FP.Open"(reference=w217, error in=w218, "State"=w216) -> (error out=w219:errorcluster)  [unwired: 2 in, 4 out]
              }
              frame False {
              }
            }
          }
        }
        n72 = call <vilib>:"Add State(s) to Queue__jki_lib_state_machine.vi"("State(s) in (\"\")"=w155) -> ("States Out"=w154:string)  [unwired: 14 in]
      }
      frame "---------- Macro ----------" {
        # "Do not put any code in this frame.\n(It is a separator no-op. You can make a copy of this frame to create a new Macro frame)"
        n73 = call <vilib>:"Add State(s) to Queue__jki_lib_state_machine.vi"("State(s) in (\"\")"=w224) -> ("States Out"=w223:string)  [unwired: 14 in]
      }
      frame "Macro: Initialize" {
        # "Initialization Macro\n(This is called once, when the VI starts)"
        n74 = call <vilib>:"Add State(s) to Queue__jki_lib_state_machine.vi"("State(s) in Front (\"\")"="Data: Initialize\nInitialize Core Data\nUI: Initialize\nUI: Front Panel State >> Open\nMacro: Test", "State(s) in (\"\")"=w229) -> ("States Out"=w228:string)  [unwired: 13 in]
      }
      frame "Macro: Test" {
        # "#Test Macro - Add the sequence \nfor measurments and limits testing here"
        n75 = call <vilib>:"Add State(s) to Queue__jki_lib_state_machine.vi"("State(s) in Front (\"\")"="Limits Test: Read Limits File\nInit: Switch Contactor", "State(s) in (\"\")"=w234) -> ("States Out"=w233:string)  [unwired: 13 in]
      }
      frame "Macro: Limits" {
        # "Do not put any code in this frame.\n(It is a separator no-op. You can make a copy of this frame to create a new Macro frame)"
        n76 = call <vilib>:"Add State(s) to Queue__jki_lib_state_machine.vi"("State(s) in Front (\"\")"="Limits Test: Connect Fail Test\nLimits Test: Connect Test\nLimits Test: UDP Read Test\nLimits Test: 5A Read Test\nLimits Test: Read ROV A Test\nLimits Test: Read ROV B Test\nLimits Test: Read TMS Test\nLimits Test: Read Wait for Start Test\nLimits Test: Read Normal Operation Test\nResults Data: Write Results Data\nMacro: Exit", "State(s) in (\"\")"=w239) -> ("States Out"=w238:string)  [unwired: 13 in]
      }
      frame "Macro: Exit" {
        # "Exit Macro\n(This is called once, when the VI exits)"
        n77 = Unbundle By Name(w246) -> ("Core.Close Panel on Exit?"=w241:bool)
        n78 = call <vilib>:"Conditional State String__jki_lib_state_machine.vi"("Do State(s)?"=w241, "State"="UI: Front Panel State >> Close") -> ("State Out"=w240:string)  [unwired: 7 in]
        n79 = call <vilib>:"Add State(s) to Queue__jki_lib_state_machine.vi"("State(s) in (\"\")"=w240, "State(s) at Back (\"\")"="UI: Uninitialize\nData: Cleanup\nExit") -> ("States Out"=w244:string)  [unwired: 13 in]
        n80 = call <vilib>:"Add State(s) to Queue__jki_lib_state_machine.vi"("State(s) in Front (\"\")"=w244, "State(s) in (\"\")"=w248) -> ("States Out"=w247:string)  [unwired: 13 in]
      }
      frame "---------- Limits Test ----------" {
        # "Template Separator\n(You can make a copy of, or modify, this frame)"
        n81 = call <vilib>:"Add State(s) to Queue__jki_lib_state_machine.vi"("State(s) in (\"\")"=w252) -> ("States Out"=w251:string)  [unwired: 14 in]
      }
      frame "Limits Test: Read Limits File" {
        w258 = ","  # delimiter (\t)
        n82 = Unbundle By Name(w255) -> ("Limits File Path"=w259:path)
        n83 = Current VI's Path "Test Case Path"() -> (path=w263:path)
        n84 = call-poly <vilib>:"Read Delimited Spreadsheet.vi"("file path (dialog if empty)"=w259, "error in (no error)"=w260, "delimiter (\\t)"=w258) -> ("all rows"=w256:string[][], "error out"=w261:errorcluster)  [unwired: 7 in, 4 out]
        n85 = Strip Path(path=w263) -> (name=w262:string)  [unwired: 1 out]
        n86 = call-poly <userlib>:"Strip Path Extension__ogtk.vi"("path"=w262) -> ("root"=w257:string)  [unwired: 1 out]
        n87 = for {
          tunnel: w257 -> [w269]
          tunnel: w256 -> [w267] mode=indexing
          tunnel: [w267] -> w253 mode=indexing if=w266
          n88 = Index Array(array=w267) -> (element=w268:string)  [unwired: 1 in]
          n89 = Equal?(x=w269, y=w268) -> (x = y?=w266:bool)
        }
        n90 = Bundle By Name(cluster=w255, "Test Limits"=w253) -> (w254:T5)
        n91 = call <vilib>:"Add State(s) to Queue__jki_lib_state_machine.vi"("State(s) in (\"\")"=w265) -> ("States Out"=w264:string)  [unwired: 14 in]
      }
      frame "Limits Test: Connect Fail Test" {
        w275 = "Connect Fail Test"  # Sub Test Name
        # "UDP Read Test = if equal to F0 = pass else fail"
        # "#Limits Testing - Add the sub test name for\ntest included in limits file"
        n92 = Unbundle By Name(w274) -> ("Test Limits"=w276:string[][], "Connect Fail"=w280:string)
        n93 = Unbundle By Name(w274) -> ("Results Data Array"=w272:string[][])
        n94 = To Variant(anything=w280) -> (Variant=w277:variant)
        n95 = call "Process Results.vi"("error in (no error)"=w278, "Measurement"=w277, "Test Limits"=w276, "Sub Test Name"=w275) -> ("error out"=w279:errorcluster, "Results Data"=w270:string[])  [unwired: 6 in]
        "Results Data 4" <- w270
        n96 = Build Array (concatenate)(w272, w270) -> (w271:string[][])
        n97 = Bundle By Name(cluster=w274, "Results Data Array"=w271) -> (w273:T5)
        n98 = call <vilib>:"Add State(s) to Queue__jki_lib_state_machine.vi"("State(s) in (\"\")"=w282) -> ("States Out"=w281:string)  [unwired: 14 in]
      }
      frame "Limits Test: Connect Test" {
        w288 = "Connect Test"  # Sub Test Name
        # "UDP Read Test = if equal to F0 = pass else fail"
        # "#Limits Testing - Add the sub test name for\ntest included in limits file"
        n99 = Unbundle By Name(w287) -> ("Results Data Array"=w285:string[][])
        n100 = Unbundle By Name(w287) -> ("Test Limits"=w289:string[][], "Connect"=w293:string)
        n101 = To Variant(anything=w293) -> (Variant=w290:variant)
        n102 = call "Process Results.vi"("error in (no error)"=w291, "Measurement"=w290, "Test Limits"=w289, "Sub Test Name"=w288) -> ("error out"=w292:errorcluster, "Results Data"=w283:string[])  [unwired: 6 in]
        "Results Data 5" <- w283
        n103 = Build Array (concatenate)(w285, w283) -> (w284:string[][])
        n104 = Bundle By Name(cluster=w287, "Results Data Array"=w284) -> (w286:T5)
        n105 = call <vilib>:"Add State(s) to Queue__jki_lib_state_machine.vi"("State(s) in (\"\")"=w295) -> ("States Out"=w294:string)  [unwired: 14 in]
      }
      frame "Limits Test: UDP Read Test" {
        w301 = "UDP Read Test"  # Sub Test Name
        # "UDP Read Test = if equal to F0 = pass else fail"
        # "#Limits Testing - Add the sub test name for\ntest included in limits file"
        n106 = Unbundle By Name(w300) -> ("Results Data Array"=w298:string[][])
        n107 = Unbundle By Name(w300) -> ("Test Limits"=w302:string[][], "UDP Read"=w306:string)
        n108 = To Variant(anything=w306) -> (Variant=w303:variant)
        n109 = call "Process Results.vi"("error in (no error)"=w304, "Measurement"=w303, "Test Limits"=w302, "Sub Test Name"=w301) -> ("error out"=w305:errorcluster, "Results Data"=w296:string[])  [unwired: 6 in]
        "Results Data 2" <- w296
        n110 = Build Array (concatenate)(w298, w296) -> (w297:string[][])
        n111 = Bundle By Name(cluster=w300, "Results Data Array"=w297) -> (w299:T5)
        n112 = call <vilib>:"Add State(s) to Queue__jki_lib_state_machine.vi"("State(s) in (\"\")"=w308) -> ("States Out"=w307:string)  [unwired: 14 in]
      }
      frame "Limits Test: 5A Read Test" {
        w314 = "5A Read Test"  # Sub Test Name
        # "UDP Read Test = if equal to F0 = pass else fail"
        # "#Limits Testing - Add the sub test name for\ntest included in limits file"
        n113 = Unbundle By Name(w313) -> ("Results Data Array"=w311:string[][])
        n114 = Unbundle By Name(w313) -> ("Test Limits"=w315:string[][], "5A Test"=w319:bool)
        n115 = To Variant(anything=w319) -> (Variant=w316:variant)
        n116 = call "Process Results.vi"("error in (no error)"=w317, "Measurement"=w316, "Test Limits"=w315, "Sub Test Name"=w314) -> ("error out"=w318:errorcluster, "Results Data"=w309:string[])  [unwired: 6 in]
        "Results Data 3" <- w309
        n117 = Build Array (concatenate)(w311, w309) -> (w310:string[][])
        n118 = Bundle By Name(cluster=w313, "Results Data Array"=w310) -> (w312:T5)
        n119 = call <vilib>:"Add State(s) to Queue__jki_lib_state_machine.vi"("State(s) in (\"\")"=w321) -> ("States Out"=w320:string)  [unwired: 14 in]
      }
      frame "Limits Test: Read ROV A Test" {
        w327 = "Read ROV A Test"  # Sub Test Name
        # "UDP Read Test = if equal to F0 = pass else fail"
        # "#Limits Testing - Add the sub test name for\ntest included in limits file"
        n120 = Unbundle By Name(w326) -> ("Test Limits"=w328:string[][], "Read ROV A"=w332:string)
        n121 = Unbundle By Name(w326) -> ("Results Data Array"=w324:string[][])
        n122 = To Variant(anything=w332) -> (Variant=w329:variant)
        n123 = call "Process Results.vi"("error in (no error)"=w330, "Measurement"=w329, "Test Limits"=w328, "Sub Test Name"=w327) -> ("error out"=w331:errorcluster, "Results Data"=w322:string[])  [unwired: 6 in]
        "Results Data 6" <- w322
        n124 = Build Array (concatenate)(w324, w322) -> (w323:string[][])
        n125 = Bundle By Name(cluster=w326, "Results Data Array"=w323) -> (w325:T5)
        n126 = call <vilib>:"Add State(s) to Queue__jki_lib_state_machine.vi"("State(s) in (\"\")"=w334) -> ("States Out"=w333:string)  [unwired: 14 in]
      }
      frame "Limits Test: Read ROV B Test" {
        w340 = "Read ROV B Test"  # Sub Test Name
        # "UDP Read Test = if equal to F0 = pass else fail"
        # "#Limits Testing - Add the sub test name for\ntest included in limits file"
        n127 = Unbundle By Name(w339) -> ("Test Limits"=w341:string[][], "Read ROV B"=w345:string)
        n128 = Unbundle By Name(w339) -> ("Results Data Array"=w337:string[][])
        n129 = To Variant(anything=w345) -> (Variant=w342:variant)
        n130 = call "Process Results.vi"("error in (no error)"=w343, "Measurement"=w342, "Test Limits"=w341, "Sub Test Name"=w340) -> ("error out"=w344:errorcluster, "Results Data"=w335:string[])  [unwired: 6 in]
        "Results Data 7" <- w335
        n131 = Build Array (concatenate)(w337, w335) -> (w336:string[][])
        n132 = Bundle By Name(cluster=w339, "Results Data Array"=w336) -> (w338:T5)
        n133 = call <vilib>:"Add State(s) to Queue__jki_lib_state_machine.vi"("State(s) in (\"\")"=w347) -> ("States Out"=w346:string)  [unwired: 14 in]
      }
      frame "Limits Test: Read TMS Test" {
        w353 = "Read TMS Test"  # Sub Test Name
        # "UDP Read Test = if equal to F0 = pass else fail"
        # "#Limits Testing - Add the sub test name for\ntest included in limits file"
        n134 = Unbundle By Name(w352) -> ("Results Data Array"=w350:string[][])
        n135 = Unbundle By Name(w352) -> ("Test Limits"=w354:string[][], "Read TMS"=w358:string)
        n136 = To Variant(anything=w358) -> (Variant=w355:variant)
        n137 = call "Process Results.vi"("error in (no error)"=w356, "Measurement"=w355, "Test Limits"=w354, "Sub Test Name"=w353) -> ("error out"=w357:errorcluster, "Results Data"=w348:string[])  [unwired: 6 in]
        "Results Data 8" <- w348
        n138 = Build Array (concatenate)(w350, w348) -> (w349:string[][])
        n139 = Bundle By Name(cluster=w352, "Results Data Array"=w349) -> (w351:T5)
        n140 = call <vilib>:"Add State(s) to Queue__jki_lib_state_machine.vi"("State(s) in (\"\")"=w360) -> ("States Out"=w359:string)  [unwired: 14 in]
      }
      frame "Limits Test: Read Wait for Start Test" {
        w366 = "Read Wait for Start Test"  # Sub Test Name
        # "UDP Read Test = if equal to F0 = pass else fail"
        # "#Limits Testing - Add the sub test name for\ntest included in limits file"
        n141 = Unbundle By Name(w365) -> ("Test Limits"=w367:string[][], "Read Wait for Start"=w371:string)
        n142 = Unbundle By Name(w365) -> ("Results Data Array"=w363:string[][])
        n143 = To Variant(anything=w371) -> (Variant=w368:variant)
        n144 = call "Process Results.vi"("error in (no error)"=w369, "Measurement"=w368, "Test Limits"=w367, "Sub Test Name"=w366) -> ("error out"=w370:errorcluster, "Results Data"=w361:string[])  [unwired: 6 in]
        "Results Data 9" <- w361
        n145 = Build Array (concatenate)(w363, w361) -> (w362:string[][])
        n146 = Bundle By Name(cluster=w365, "Results Data Array"=w362) -> (w364:T5)
        n147 = call <vilib>:"Add State(s) to Queue__jki_lib_state_machine.vi"("State(s) in (\"\")"=w373) -> ("States Out"=w372:string)  [unwired: 14 in]
      }
      frame "Limits Test: Read Normal Operation Test" {
        w379 = "Read Normal Operation Test"  # Sub Test Name
        # "UDP Read Test = if equal to F0 = pass else fail"
        # "#Limits Testing - Add the sub test name for\ntest included in limits file"
        n148 = Unbundle By Name(w378) -> ("Test Limits"=w380:string[][], "Read Normal Operation"=w384:string)
        n149 = Unbundle By Name(w378) -> ("Results Data Array"=w376:string[][])
        n150 = To Variant(anything=w384) -> (Variant=w381:variant)
        n151 = call "Process Results.vi"("error in (no error)"=w382, "Measurement"=w381, "Test Limits"=w380, "Sub Test Name"=w379) -> ("error out"=w383:errorcluster, "Results Data"=w374:string[])  [unwired: 6 in]
        "Results Data 10" <- w374
        n152 = Build Array (concatenate)(w376, w374) -> (w375:string[][])
        n153 = Bundle By Name(cluster=w378, "Results Data Array"=w375) -> (w377:T5)
        n154 = call <vilib>:"Add State(s) to Queue__jki_lib_state_machine.vi"("State(s) in (\"\")"=w386) -> ("States Out"=w385:string)  [unwired: 14 in]
      }
      frame "---------- Results Data ----------" {
        # "Template Separator\n(You can make a copy of, or modify, this frame)"
        n155 = call <vilib>:"Add State(s) to Queue__jki_lib_state_machine.vi"("State(s) in (\"\")"=w390) -> ("States Out"=w389:string)  [unwired: 14 in]
      }
      frame "Results Data: Write Results Data" {
        w392 = ","  # delimiter (\t)
        w393 = TRUE  # append to file? (new file:F)
        n156 = Unbundle By Name(w395) -> ("Results File Path"=w394:path, "Results Data Array"=w391:string[][])
        "Results Data Array" <- w391
        n157 = call-poly <vilib>:"Write Delimited Spreadsheet.vi"("file path (dialog if empty)"=w394, "2D data"=w391, "append to file? (new file:F)"=w393, "error in (no error)"=w396, "delimiter (\\t)"=w392) -> ("error out"=w397:errorcluster)  [unwired: 9 in, 1 out]
        n158 = call <vilib>:"Add State(s) to Queue__jki_lib_state_machine.vi"("State(s) in (\"\")"=w399) -> ("States Out"=w398:string)  [unwired: 14 in]
      }
      frame "---------- Init ----------" {
        # "Template Separator\n(You can make a copy of, or modify, this frame)"
        n159 = call <vilib>:"Add State(s) to Queue__jki_lib_state_machine.vi"("State(s) in (\"\")"=w403) -> ("States Out"=w402:string)  [unwired: 14 in]
      }
      frame "Init: Switch Contactor" {
        # "Template Separator\n(You can make a copy of, or modify, this frame)"
        # "User must set IP address to match this given one"
        n160 = call-poly <vilib>:"DAQmx Create Virtual Channel.vi"("lines"=tag "6525/port0/line0", "error in"=w412) -> ("task out"=w415:refnum<k21>, "error out"=w414:errorcluster)  [unwired: 12 in]
        n161 = call <vilib>:"DAQmx Start Task.vi"("task/channels in"=w415, "error in"=w414) -> ("task out"=w410:refnum<k21>, "error out"=w411:errorcluster)  [unwired: 12 in]
        n162 = call-poly <vilib>:"DAQmx Write.vi"("task/channels in"=w410, "data"=bool[] [TRUE], "error in"=w411) -> ("task out"=w405:refnum<k21>, "error out"=w409:errorcluster)  [unwired: 10 in, 1 out]
        n163 = call <vilib>:"DAQmx Stop Task.vi"("task/channels in"=w405, "error in"=w409) -> ("task out"=w406:refnum<k21>, "error out"=w408:errorcluster)  [unwired: 12 in]
        n164 = call <vilib>:"DAQmx Clear Task.vi"("task in"=w406, "error in"=w408) -> ("error out"=w407:errorcluster)  [unwired: 13 in]
        n165 = call <vilib>:"Add State(s) to Queue__jki_lib_state_machine.vi"("State(s) in Front (\"\")"="Init: Set IP Address" ("State(s) in Front (\"\")"), "State(s) in (\"\")"=w419) -> ("States Out"=w418:string)  [unwired: 13 in]
      }
      frame "Init: Set IP Address" {
        # "Template Separator\n(You can make a copy of, or modify, this frame)"
        # "User must set IP address to match this given one"
        n166 = One Button Dialog(message="Make your IP Address 192.168.201.22", button name ("OK")="Done") -> ()  [unwired: 1 out]
        n167 = call <vilib>:"Add State(s) to Queue__jki_lib_state_machine.vi"("State(s) in Front (\"\")"="Init: UDP Open" ("State(s) in Front (\"\")"), "State(s) in (\"\")"=w426) -> ("States Out"=w425:string)  [unwired: 13 in]
      }
      frame "Init: UDP Open" {
        # "If this changes \nchange on CONNECT command as well!"
        # "User must enter their PC IP address"
        # "Open UDP read to RIB box"
        # "Template Separator\n(You can make a copy of, or modify, this frame)"
        # "Open UDP linking to RIB Box."
        n168 = String To IP(1:"192.168.201.22" ("name")) -> (0:w436:u32)
        n169 = UDP Open(7:w436, 8:w435, 11:u16 54321 ("port")) -> (port=w429:refnum<k16>, 0:w431:errorcluster)  [unwired: 2 in, 1 out]
        n170 = call "FGV - Initialise.vi"("Enum"=FGV_-_Enum."Open UDP", "connection ID"=w429, "Error In"=w431) -> ("Error Out"=w430:errorcluster)  [unwired: 9 in, 3 out]
        n171 = Bundle By Name(cluster=w434, "connection ID"=w429) -> (w433:T5)
        n172 = call <vilib>:"Add State(s) to Queue__jki_lib_state_machine.vi"("State(s) in Front (\"\")"="Init: I2C Open" ("State(s) in Front (\"\")"), "State(s) in (\"\")"=w439) -> ("States Out"=w438:string)  [unwired: 13 in]
      }
      frame "Init: I2C Open" {
        # "Template Separator\n(You can make a copy of, or modify, this frame)"
        n173 = call "FGV - Initialise.vi"("Enum"=FGV_-_Enum."Get Data", "Error In"=w442) -> ("task out"=w441:refnum<k21>, "Error Out"=w443:errorcluster)  [unwired: 10 in, 2 out]
        n174 = Bundle By Name(cluster=w446, "task out"=w441) -> (w445:T5)
        n175 = call <vilib>:"Add State(s) to Queue__jki_lib_state_machine.vi"("State(s) in Front (\"\")"="Init: UPD Connect Fail" ("State(s) in Front (\"\")"), "State(s) in (\"\")"=w448) -> ("States Out"=w447:string)  [unwired: 13 in]
      }
      frame "Init: UPD Connect Fail" {
        # "Send CONNECT command to RIB Box"
        # "IP for RIB Box is set"
        # "Data"
        # "Length"
        # "ID"
        # "Target"
        # "Type"
        # "Pkt ID"
        # "CONNECT"
        # "Template Separator\n(You can make a copy of, or modify, this frame)"
        n176 = Unbundle By Name(w453) -> ("connection ID"=w452:refnum<k16>)
        n177 = Build Array(u8 91 ("element"), u8 1 ("element"), u8 9 ("element"), u8 1 ("element"), u8 5 ("element"), u8 192 ("element"), u8 168 ("element"), u8 201 ("element"), u8 255 ("element")) -> (w468:u8[])
        n178 = Byte Array To String(unsigned byte array=w468) -> (string=w469:string)
        n179 = String To IP(1:"192.168.201.21" ("name")) -> (0:w457:u32)
        n180 = UDP Write(address=w457, port or service name=u16 54321, connection ID=w452, data in=w469, 8:w454, 9:1000 ("timeout ms (25000)")) -> (error out=w449:errorcluster, 3:w451:refnum<k16>)
        n181 = Bundle By Name(cluster=w453, "connection ID"=w451) -> (w455:T5)
        n182 = call <vilib>:"Add State(s) to Queue__jki_lib_state_machine.vi"("State(s) in Front (\"\")"="Init: Read Connect Fail" ("State(s) in Front (\"\")"), "State(s) in (\"\")"=w472) -> ("States Out"=w471:string)  [unwired: 13 in]
      }
      frame "Init: Read Connect Fail" {
        # "Read UDP if equal to F0 test complete if not check if timer has elapsed."
        # "#56 = didnt read before the timeout"
        # "Template Separator\n(You can make a copy of, or modify, this frame)"
        n183 = Unbundle By Name(w485) -> ("connection ID"=w486:refnum<k16>)
        n184 = UDP Read(connection ID=w486, timeout ms (25000)=10, 8:w487) -> (data out=w474:string, error out=w479:errorcluster, 3:w476:refnum<k16>)  [unwired: 1 in, 2 out]
        n185 = String To Byte Array(string=w474) -> (unsigned byte array=w483:u8[])
        n186 = Number To Hexadecimal String(2:w483) -> (0:w482:string[])  [unwired: 1 in]
        n187 = Index Array(array=w482, index=0) -> (element=w473:string)
        "Connect Fail" <- w473
        n188 = call <vilib>:"Clear Errors.vi"("error in (no error)"=w479, "specific error code to clear (0: all)"=56) -> ("error out"=w478:errorcluster)  [unwired: 4 in, 1 out]
        n189 = Bundle By Name(cluster=w485, "connection ID"=w476, "Connect Fail"=w473) -> (w484:T5)
        n190 = call <vilib>:"Add State(s) to Queue__jki_lib_state_machine.vi"("State(s) in Front (\"\")"="Init: UPD Connect" ("State(s) in Front (\"\")"), "State(s) in (\"\")"=w489) -> ("States Out"=w488:string)  [unwired: 13 in]
      }
      frame "Init: UPD Connect" {
        # "Length Wrong to froce a fail!"
        # "Send CONNECT command to RIB Box"
        # "IP for RIB Box is set"
        # "Data"
        # "Length"
        # "ID"
        # "Target"
        # "Type"
        # "Pkt ID"
        # "CONNECT"
        # "Template Separator\n(You can make a copy of, or modify, this frame)"
        n191 = Unbundle By Name(w494) -> ("connection ID"=w493:refnum<k16>)
        n192 = Build Array(u8 91 ("element"), u8 1 ("element"), u8 9 ("element"), u8 1 ("element"), u8 4 ("element"), u8 192 ("element"), u8 168 ("element"), u8 201 ("element"), u8 22 ("element")) -> (w509:u8[])
        n193 = Byte Array To String(unsigned byte array=w509) -> (string=w510:string)
        n194 = String To IP(1:"192.168.201.21" ("name")) -> (0:w498:u32)
        n195 = UDP Write(address=w498, port or service name=u16 54321, connection ID=w493, data in=w510, 8:w495, 9:1000 ("timeout ms (25000)")) -> (error out=w490:errorcluster, 3:w492:refnum<k16>)
        n196 = Bundle By Name(cluster=w494, "connection ID"=w492) -> (w496:T5)
        n197 = call <vilib>:"Add State(s) to Queue__jki_lib_state_machine.vi"("State(s) in Front (\"\")"="Init: Read Connect" ("State(s) in Front (\"\")"), "State(s) in (\"\")"=w513) -> ("States Out"=w512:string)  [unwired: 13 in]
      }
      frame "Init: Read Connect" {
        # "Read UDP if equal to F0 test complete if not check if timer has elapsed."
        # "#56 = didnt read before the timeout"
        # "Template Separator\n(You can make a copy of, or modify, this frame)"
        n198 = Unbundle By Name(w526) -> ("connection ID"=w527:refnum<k16>)
        n199 = UDP Read(connection ID=w527, timeout ms (25000)=10, 8:w528) -> (data out=w515:string, error out=w523:errorcluster, 3:w520:refnum<k16>)  [unwired: 1 in, 2 out]
        n200 = String To Byte Array(string=w515) -> (unsigned byte array=w518:u8[])
        n201 = Number To Hexadecimal String(2:w518) -> (0:w517:string[])  [unwired: 1 in]
        n202 = Index Array(array=w517, index=0) -> (element=w514:string)
        "Connect" <- w514
        n203 = call <vilib>:"Clear Errors.vi"("error in (no error)"=w523, "specific error code to clear (0: all)"=56) -> ("error out"=w522:errorcluster)  [unwired: 4 in, 1 out]
        n204 = Bundle By Name(cluster=w526, "connection ID"=w520, "Connect"=w514) -> (w525:T5)
        n205 = call <vilib>:"Add State(s) to Queue__jki_lib_state_machine.vi"("State(s) in Front (\"\")"="Init: Start Timer" ("State(s) in Front (\"\")"), "State(s) in (\"\")"=w530) -> ("States Out"=w529:string)  [unwired: 13 in]
      }
      frame "Init: Start Timer" {
        # "Start 10 second timer"
        # "Template Separator\n(You can make a copy of, or modify, this frame)"
        n206 = call "Timer.vi"("error in (no error)"=w537, "Enum"=T4."Start Timer") -> ("error out"=w536:errorcluster)  [unwired: 6 in, 3 out]
        n207 = property on="Timeout (Read UDP)" class="Slide (strict)"(error in=w536, "Value"=0.0 ("Horizontal Pointer Slide"), "Scale.Maximum"=20.0 ("Target Time"), "Scale.Minimum"=0.0 ("Scale.Range:Minimum")) -> (error out=w532:errorcluster)  [unwired: 1 in, 1 out]
        n208 = call <vilib>:"Add State(s) to Queue__jki_lib_state_machine.vi"("State(s) in Front (\"\")"="Init: UPD Enable UPS" ("State(s) in Front (\"\")"), "State(s) in (\"\")"=w541) -> ("States Out"=w540:string)  [unwired: 13 in]
      }
      frame "Init: UPD Enable UPS" {
        # "Send Enable UPS command to RIB Box"
        # "ENABLE UPS"
        # "Template Separator\n(You can make a copy of, or modify, this frame)"
        n209 = Unbundle By Name(w545) -> ("connection ID"=w544:refnum<k16>)
        n210 = Build Array(u8 91 ("element"), u8 1 ("element"), u8 9 ("element"), u8 112 ("element"), u8 1 ("element"), u8 1 ("element")) -> (w559:u8[])
        n211 = String To IP(1:"192.168.201.21" ("name")) -> (0:w552:u32)
        n212 = Byte Array To String(unsigned byte array=w559) -> (string=w553:string)
        n213 = UDP Write(address=w552, port or service name=u16 54321, connection ID=w544, data in=w553, 8:w547, 9:1000 ("timeout ms (25000)")) -> (error out=w542:errorcluster, 3:w548:refnum<k16>)
        n214 = Bundle By Name(cluster=w545, "connection ID"=w548) -> (w549:T5)
        n215 = call <vilib>:"Add State(s) to Queue__jki_lib_state_machine.vi"("State(s) in Front (\"\")"="Init: Read UDP" ("State(s) in Front (\"\")"), "State(s) in (\"\")"=w562) -> ("States Out"=w561:string)  [unwired: 13 in]
      }
      frame "Init: Read UDP" {
        # "Read UDP if equal to F0 test complete if not check if timer has elapsed."
        # "#56 = didnt read before the timeout"
        # "Template Separator\n(You can make a copy of, or modify, this frame)"
        n216 = Unbundle By Name(w580) -> ("connection ID"=w581:refnum<k16>)
        n217 = UDP Read(connection ID=w581, timeout ms (25000)=10, 8:w582) -> (data out=w568:string, error out=w567:errorcluster, 3:w563:refnum<k16>)  [unwired: 1 in, 2 out]
        n218 = String Subset(string=w568, offset (0)=81 ("offset (0) 2"), length (rest)=1 ("length (rest) 2")) -> (substring=w575:string)
        n219 = String To Byte Array(string=w575) -> (unsigned byte array=w578:u8[])
        n220 = Number To Hexadecimal String(2:w578) -> (0:w577:string[])  [unwired: 1 in]
        n221 = Index Array(array=w577, index=0) -> (element=w564:string)
        n222 = call <vilib>:"Clear Errors.vi"("error in (no error)"=w567, "specific error code to clear (0: all)"=56) -> ("error out"=w566:errorcluster)  [unwired: 4 in, 1 out]
        n223 = Equal?(x=w564, y="F0") -> (x = y?=w572:bool)
        n224 = Bundle By Name(cluster=w580, "connection ID"=w563, "UDP Read"=w564) -> (w579:T5)
        n225 = call-poly <vilib>:"Select State(s)__jki_lib_state_machine.vi"("State(s) if True (\"\")"="Init: Start Timer (5A)" ("State(s) if True (\"\")"), "Select"=w572, "State(s) if False (\"\")"="Init: Elapsed Timer" ("State(s) if False (\"\")")) -> ("States Out"=w570:string)  [unwired: 12 in]
        n226 = call <vilib>:"Add State(s) to Queue__jki_lib_state_machine.vi"("State(s) in Front (\"\")"=w570, "State(s) in (\"\")"=w586) -> ("States Out"=w585:string)  [unwired: 13 in]
      }
      frame "Init: Elapsed Timer" {
        # "check if timer elased - if TRUE end test if FALSE read again."
        # "Template Separator\n(You can make a copy of, or modify, this frame)"
        # "Check to see if the timer has elpased."
        n227 = call "Timer.vi"("error in (no error)"=w594, "Target Time"=20.0, "Enum"=T4."Get Time") -> ("error out"=w593:errorcluster, "Time Elapsed?"=w590:bool, "Elapsed Time"=→"Timeout (Read UDP)":dbl)  [unwired: 5 in, 1 out]
        n228 = call-poly <vilib>:"Select State(s)__jki_lib_state_machine.vi"("State(s) if True (\"\")"="Init: Start Timer (5A)" ("State(s) if True (\"\")"), "Select"=w590, "State(s) if False (\"\")"="Init: Read UDP" ("State(s) if False (\"\")")) -> ("States Out"=w589:string)  [unwired: 12 in]
        n229 = call <vilib>:"Add State(s) to Queue__jki_lib_state_machine.vi"("State(s) in Front (\"\")"=w589, "State(s) in (\"\")"=w598) -> ("States Out"=w597:string)  [unwired: 13 in]
      }
      frame "Init: Start Timer (5A)" {
        # "Start 5 second timer"
        # "Template Separator\n(You can make a copy of, or modify, this frame)"
        n230 = call "Timer.vi"("error in (no error)"=w605, "Enum"=T4."Start Timer") -> ("error out"=w600:errorcluster)  [unwired: 6 in, 3 out]
        n231 = property on="Timeout (5A)" class="Slide (strict)"(error in=w600, "Value"=0.0 ("Horizontal Pointer Slide"), "Scale.Maximum"=5.0 ("Target Time"), "Scale.Minimum"=0.0 ("Scale.Range:Minimum")) -> (error out=w599:errorcluster)  [unwired: 1 in, 1 out]
        n232 = call <vilib>:"Add State(s) to Queue__jki_lib_state_machine.vi"("State(s) in Front (\"\")"="Init: Check 5A" ("State(s) in Front (\"\")"), "State(s) in (\"\")"=w609) -> ("States Out"=w608:string)  [unwired: 13 in]
      }
      frame "Init: Check 5A" {
        # "Template Copyright © 2024 JKI - http://jki.net/state-machine"
        # "Measure 5A from the 6525. If it can be read test complete else the timer progress is made."
        n233 = Unbundle By Name(w625) -> ("task out"=w616:refnum<k21>)
        n234 = call-poly <vilib>:"DAQmx Read.vi"("task/channels in"=w616, "error in"=w615) -> ("task out"=w610:refnum<k21>, "data"=w623:bool[], "error out"=w614:errorcluster)  [unwired: 11 in]
        n235 = Equal?(x=bool[] [TRUE, TRUE, TRUE, TRUE, FALSE], y=w623) -> (x = y?=w618:bool[])
        n236 = Array To Cluster(array=w618) -> (cluster=w619:T7)
        n237 = Unbundle(w619) -> ("[0]"=w620:bool, "[1]"=w621:bool, "[2]"=w622:bool, "[3]"=w612:bool)  [unwired: 5 out]
        n238 = Compound Arithmetic op=AND(w620, w621, w622, w612) -> (w611:bool)
        "5A Test" <- w611
        n239 = Bundle By Name(cluster=w625, "task out"=w610, "5A Test"=w611) -> (w624:T5)
        n240 = call-poly <vilib>:"Select State(s)__jki_lib_state_machine.vi"("State(s) if True (\"\")"="Init: Enable ROV A, ROV B and TMS" ("State(s) if True (\"\")"), "Select"=w611, "State(s) if False (\"\")"="Init: Elapsed Timer (5A)" ("State(s) if False (\"\")")) -> ("States Out"=w626:string)  [unwired: 12 in]
        n241 = call <vilib>:"Add State(s) to Queue__jki_lib_state_machine.vi"("State(s) in Front (\"\")"=w626, "State(s) in (\"\")"=w629) -> ("States Out"=w628:string)  [unwired: 13 in]
      }
      frame "Init: Elapsed Timer (5A)" {
        # "check if timer elased - if TRUE end test if FALSE read again."
        # "Template Separator\n(You can make a copy of, or modify, this frame)"
        n242 = call "Timer.vi"("error in (no error)"=w637, "Target Time"=5.0, "Enum"=T4."Get Time") -> ("error out"=w636:errorcluster, "Time Elapsed?"=w633:bool, "Elapsed Time"=→"Timeout (5A)":dbl)  [unwired: 5 in, 1 out]
        n243 = call-poly <vilib>:"Select State(s)__jki_lib_state_machine.vi"("State(s) if True (\"\")"="Init: Enable ROV A, ROV B and TMS" ("State(s) if True (\"\")"), "Select"=w633, "State(s) if False (\"\")"="Init: Check 5A" ("State(s) if False (\"\")")) -> ("States Out"=w632:string)  [unwired: 12 in]
        n244 = call <vilib>:"Add State(s) to Queue__jki_lib_state_machine.vi"("State(s) in Front (\"\")"=w632, "State(s) in (\"\")"=w641) -> ("States Out"=w640:string)  [unwired: 13 in]
      }
      frame "Init: Enable ROV A, ROV B and TMS" {
        w670 = u16 54321 ("port or service name")
        # "Data"
        # "Length"
        # "ID"
        # "Target"
        # "Type"
        # "Pkt ID"
        # "Data"
        # "Length"
        # "ID"
        # "Target"
        # "Type"
        # "Pkt ID"
        # "Data"
        # "Length"
        # "ID"
        # "Target"
        # "Type"
        # "Pkt ID"
        # "Send Enable UPS command to RIB Box"
        # "Template Separator\n(You can make a copy of, or modify, this frame)"
        n245 = Unbundle By Name(w650) -> ("connection ID"=w649:refnum<k16>)
        n246 = Build Array(u8 91 ("element"), u8 1 ("element"), u8 9 ("element"), u8 105 ("element"), u8 1 ("element"), u8 1 ("element")) -> (w680:u8[])
        n247 = Byte Array To String(unsigned byte array=w680) -> (string=w677:string)
        n248 = String To IP(1:"192.168.201.21" ("name")) -> (0:w683:u32)
        n249 = UDP Write(address=w683, port or service name=w670, connection ID=w649, data in=w677, 8:w653, 9:1000 ("timeout ms (25000)")) -> (error out=w642:errorcluster, 3:w646:refnum<k16>)
        n250 = Build Array(u8 91 ("element"), u8 1 ("element"), u8 9 ("element"), u8 106 ("element"), u8 1 ("element"), u8 1 ("element")) -> (w681:u8[])
        n251 = Byte Array To String(unsigned byte array=w681) -> (string=w678:string)
        n252 = UDP Write(address=w683, port or service name=w670, connection ID=w646, data in=w678, 8:w642, 9:1000 ("timeout ms (25000)")) -> (error out=w652:errorcluster, 3:w647:refnum<k16>)
        n253 = Build Array(u8 91 ("element"), u8 1 ("element"), u8 9 ("element"), u8 107 ("element"), u8 1 ("element"), u8 1 ("element")) -> (w682:u8[])
        n254 = Byte Array To String(unsigned byte array=w682) -> (string=w679:string)
        n255 = UDP Write(address=w683, port or service name=w670, connection ID=w647, data in=w679, 8:w652, 9:1000 ("timeout ms (25000)")) -> (error out=w645:errorcluster, 3:w651:refnum<k16>)
        n256 = Bundle By Name(cluster=w650, "connection ID"=w651) -> (w684:T5)
        n257 = call <userlib>:"Wait (ms)__ogtk.vi"("error in (no error)"=w645, "milliseconds to wait"=u32 1000) -> ("error out"=w644:errorcluster)  [unwired: 8 in, 1 out]
        n258 = call <vilib>:"Add State(s) to Queue__jki_lib_state_machine.vi"("State(s) in Front (\"\")"="Init: Set Command" ("State(s) in Front (\"\")"), "State(s) in (\"\")"=w686) -> ("States Out"=w685:string)  [unwired: 13 in]
      }
      frame "Init: Set Command" {
        # "RIB Box IP"
        # "Data"
        # "Length"
        # "ID"
        # "Target"
        # "Type"
        # "Pkt ID"
        # "SET"
        # "Template Separator\n(You can make a copy of, or modify, this frame)"
        n259 = Unbundle By Name(w705) -> ("connection ID"=w692:refnum<k16>)
        n260 = Build Array(u8 91 ("element"), u8 1 ("element"), u8 9 ("element"), u8 108 ("element"), u8 0 ("element")) -> (w703:u8[])
        n261 = Byte Array To String(unsigned byte array=w703) -> (string=w704:string)
        n262 = String To IP(1:"192.168.201.21" ("name")) -> (0:w696:u32)
        n263 = UDP Write(address=w696, port or service name=u16 54321, connection ID=w692, data in=w704, 8:w694, 9:1000 ("timeout ms (25000)")) -> (error out=w689:errorcluster, 3:w693:refnum<k16>)
        n264 = Bundle By Name(cluster=w705, "connection ID"=w693) -> (w706:T5)
        n265 = call <userlib>:"Wait (ms)__ogtk.vi"("error in (no error)"=w689, "milliseconds to wait"=u32 1000) -> ("error out"=w688:errorcluster)  [unwired: 8 in, 1 out]
        n266 = call <vilib>:"Add State(s) to Queue__jki_lib_state_machine.vi"("State(s) in Front (\"\")"="Init: Start Timer (ROV A)" ("State(s) in Front (\"\")"), "State(s) in (\"\")"=w708) -> ("States Out"=w707:string)  [unwired: 13 in]
      }
      frame "Init: Start Timer (ROV A)" {
        # "Start 10 second timer"
        # "Template Separator\n(You can make a copy of, or modify, this frame)"
        n267 = call "Timer.vi"("error in (no error)"=w715, "Enum"=T4."Start Timer") -> ("error out"=w714:errorcluster)  [unwired: 6 in, 3 out]
        n268 = property on="Timeout (Read States)" class="Slide (strict)"(error in=w714, "Value"=0.0 ("Horizontal Pointer Slide"), "Scale.Maximum"=15.0 ("Target Time"), "Scale.Minimum"=0.0 ("Scale.Range:Minimum")) -> (error out=w710:errorcluster)  [unwired: 1 in, 1 out]
        n269 = call <vilib>:"Add State(s) to Queue__jki_lib_state_machine.vi"("State(s) in Front (\"\")"="Init: Read ROV A State" ("State(s) in Front (\"\")"), "State(s) in (\"\")"=w719) -> ("States Out"=w718:string)  [unwired: 13 in]
      }
      frame "Init: Read ROV A State" {
        # "Read UDP if equal to F0 test complete if not check if timer has elapsed."
        # "#56 = didnt read before the timeout"
        # "Template Separator\n(You can make a copy of, or modify, this frame)"
        n270 = Unbundle By Name(w729) -> ("connection ID"=w739:refnum<k16>)
        n271 = UDP Read(connection ID=w739, timeout ms (25000)=1, 8:w726) -> (data out=w733:string, error out=w732:errorcluster, 3:w730:refnum<k16>)  [unwired: 1 in, 2 out]
        n272 = String Subset(string=w733, offset (0)=17 ("offset (0) 2"), length (rest)=1 ("length (rest) 2")) -> (substring=w735:string)
        n273 = String To Byte Array(string=w735) -> (unsigned byte array=w738:u8[])
        n274 = Number To Hexadecimal String(2:w738) -> (0:w737:string[])  [unwired: 1 in]
        n275 = Index Array(array=w737, index=0) -> (element=w720:string)
        "element" <- w720
        n276 = Equal?(x=w720, y="C") -> (x = y?=w721:bool)
        "ROV A Enabled" <- w721
        n277 = call <vilib>:"Clear Errors.vi"("error in (no error)"=w732, "specific error code to clear (0: all)"=56) -> ("error out"=w727:errorcluster)  [unwired: 4 in, 1 out]
        n278 = Bundle By Name(cluster=w729, "connection ID"=w730, "Read ROV A"=w720) -> (w728:T5)
        n279 = call-poly <vilib>:"Select State(s)__jki_lib_state_machine.vi"("State(s) if True (\"\")"="Init: Start Timer (ROV B)" ("State(s) if True (\"\")"), "Select"=w721, "State(s) if False (\"\")"="Init: Elapsed Timer (ROV A)" ("State(s) if False (\"\")")) -> ("States Out"=w722:string)  [unwired: 12 in]
        n280 = call <vilib>:"Add State(s) to Queue__jki_lib_state_machine.vi"("State(s) in Front (\"\")"=w722, "State(s) in (\"\")"=w743) -> ("States Out"=w742:string)  [unwired: 13 in]
      }
      frame "Init: Elapsed Timer (ROV A)" {
        # "check if timer elased - if TRUE end test if FALSE read again."
        # "Template Separator\n(You can make a copy of, or modify, this frame)"
        # "Check to see if the timer has elpased."
        n281 = call "Timer.vi"("error in (no error)"=w751, "Target Time"=15.0, "Enum"=T4."Get Time") -> ("error out"=w750:errorcluster, "Time Elapsed?"=w747:bool, "Elapsed Time"=→"Timeout (Read States)":dbl)  [unwired: 5 in, 1 out]
        n282 = call-poly <vilib>:"Select State(s)__jki_lib_state_machine.vi"("State(s) if True (\"\")"="Init: Start Timer (ROV B)" ("State(s) if True (\"\")"), "Select"=w747, "State(s) if False (\"\")"="Init: Read ROV A State" ("State(s) if False (\"\")")) -> ("States Out"=w746:string)  [unwired: 12 in]
        n283 = call <vilib>:"Add State(s) to Queue__jki_lib_state_machine.vi"("State(s) in Front (\"\")"=w746, "State(s) in (\"\")"=w755) -> ("States Out"=w754:string)  [unwired: 13 in]
      }
      frame "Init: Start Timer (ROV B)" {
        # "Start 10 second timer"
        # "Template Separator\n(You can make a copy of, or modify, this frame)"
        n284 = call "Timer.vi"("error in (no error)"=w762, "Enum"=T4."Start Timer") -> ("error out"=w761:errorcluster)  [unwired: 6 in, 3 out]
        n285 = property on="Timeout (Read States) 2" class="Slide (strict)"(error in=w761, "Value"=0.0 ("Horizontal Pointer Slide"), "Scale.Maximum"=10.0 ("Target Time"), "Scale.Minimum"=0.0 ("Scale.Range:Minimum")) -> (error out=w757:errorcluster)  [unwired: 1 in, 1 out]
        n286 = call <vilib>:"Add State(s) to Queue__jki_lib_state_machine.vi"("State(s) in Front (\"\")"="Init: Read ROV B State" ("State(s) in Front (\"\")"), "State(s) in (\"\")"=w766) -> ("States Out"=w765:string)  [unwired: 13 in]
      }
      frame "Init: Read ROV B State" {
        # "Read UDP if equal to F0 test complete if not check if timer has elapsed."
        # "#56 = didnt read before the timeout"
        # "Template Separator\n(You can make a copy of, or modify, this frame)"
        n287 = Unbundle By Name(w773) -> ("connection ID"=w786:refnum<k16>)
        n288 = UDP Read(connection ID=w786, timeout ms (25000)=1, 8:w768) -> (data out=w780:string, error out=w779:errorcluster, 3:w770:refnum<k16>)  [unwired: 1 in, 2 out]
        n289 = String Subset(string=w780, offset (0)=17 ("offset (0) 2"), length (rest)=1 ("length (rest) 2")) -> (substring=w782:string)
        n290 = String To Byte Array(string=w782) -> (unsigned byte array=w785:u8[])
        n291 = Number To Hexadecimal String(2:w785) -> (0:w784:string[])  [unwired: 1 in]
        n292 = Index Array(array=w784, index=0) -> (element=w774:string)
        n293 = Equal?(x=w774, y="F") -> (x = y?=w767:bool)
        "ROV B Enabled" <- w767
        n294 = call <vilib>:"Clear Errors.vi"("error in (no error)"=w779, "specific error code to clear (0: all)"=56) -> ("error out"=w769:errorcluster)  [unwired: 4 in, 1 out]
        n295 = Bundle By Name(cluster=w773, "connection ID"=w770, "Read ROV B"=w774) -> (w772:T5)
        n296 = call-poly <vilib>:"Select State(s)__jki_lib_state_machine.vi"("State(s) if True (\"\")"="Init: Start Timer (TMS)" ("State(s) if True (\"\")"), "Select"=w767, "State(s) if False (\"\")"="Init: Elapsed Timer (ROV B)" ("State(s) if False (\"\")")) -> ("States Out"=w771:string)  [unwired: 12 in]
        n297 = call <vilib>:"Add State(s) to Queue__jki_lib_state_machine.vi"("State(s) in Front (\"\")"=w771, "State(s) in (\"\")"=w790) -> ("States Out"=w789:string)  [unwired: 13 in]
      }
      frame "Init: Elapsed Timer (ROV B)" {
        # "check if timer elased - if TRUE end test if FALSE read again."
        # "Template Separator\n(You can make a copy of, or modify, this frame)"
        # "Check to see if the timer has elpased."
        n298 = call "Timer.vi"("error in (no error)"=w798, "Target Time"=10.0, "Enum"=T4."Get Time") -> ("error out"=w797:errorcluster, "Time Elapsed?"=w794:bool, "Elapsed Time"=→"Timeout (Read States) 2":dbl)  [unwired: 5 in, 1 out]
        n299 = call-poly <vilib>:"Select State(s)__jki_lib_state_machine.vi"("State(s) if True (\"\")"="Init: Start Timer (TMS)" ("State(s) if True (\"\")"), "Select"=w794, "State(s) if False (\"\")"="Init: Read ROV B State" ("State(s) if False (\"\")")) -> ("States Out"=w793:string)  [unwired: 12 in]
        n300 = call <vilib>:"Add State(s) to Queue__jki_lib_state_machine.vi"("State(s) in Front (\"\")"=w793, "State(s) in (\"\")"=w802) -> ("States Out"=w801:string)  [unwired: 13 in]
      }
      frame "Init: Start Timer (TMS)" {
        # "Start 10 second timer"
        # "Template Separator\n(You can make a copy of, or modify, this frame)"
        n301 = call "Timer.vi"("error in (no error)"=w809, "Enum"=T4."Start Timer") -> ("error out"=w808:errorcluster)  [unwired: 6 in, 3 out]
        n302 = property on="Timeout (Read States) 3" class="Slide (strict)"(error in=w808, "Value"=0.0 ("Horizontal Pointer Slide"), "Scale.Maximum"=10.0 ("Target Time"), "Scale.Minimum"=0.0 ("Scale.Range:Minimum")) -> (error out=w804:errorcluster)  [unwired: 1 in, 1 out]
        n303 = call <vilib>:"Add State(s) to Queue__jki_lib_state_machine.vi"("State(s) in Front (\"\")"="Init: Read TMS State" ("State(s) in Front (\"\")"), "State(s) in (\"\")"=w813) -> ("States Out"=w812:string)  [unwired: 13 in]
      }
      frame "Init: Read TMS State" {
        # "Read UDP if equal to F0 test complete if not check if timer has elapsed."
        # "#56 = didnt read before the timeout"
        # "Template Separator\n(You can make a copy of, or modify, this frame)"
        n304 = Unbundle By Name(w820) -> ("connection ID"=w833:refnum<k16>)
        n305 = UDP Read(connection ID=w833, timeout ms (25000)=1, 8:w815) -> (data out=w827:string, error out=w826:errorcluster, 3:w817:refnum<k16>)  [unwired: 1 in, 2 out]
        n306 = String Subset(string=w827, offset (0)=17 ("offset (0) 2"), length (rest)=1 ("length (rest) 2")) -> (substring=w829:string)
        n307 = String To Byte Array(string=w829) -> (unsigned byte array=w832:u8[])
        n308 = Number To Hexadecimal String(2:w832) -> (0:w831:string[])  [unwired: 1 in]
        n309 = Index Array(array=w831, index=0) -> (element=w821:string)
        n310 = Equal?(x=w821, y="12") -> (x = y?=w814:bool)
        "TMS Enabled" <- w814
        n311 = call <vilib>:"Clear Errors.vi"("error in (no error)"=w826, "specific error code to clear (0: all)"=56) -> ("error out"=w816:errorcluster)  [unwired: 4 in, 1 out]
        n312 = Bundle By Name(cluster=w820, "connection ID"=w817, "Read TMS"=w821) -> (w819:T5)
        n313 = call-poly <vilib>:"Select State(s)__jki_lib_state_machine.vi"("State(s) if True (\"\")"="Init: Start Timer (WfS)" ("State(s) if True (\"\")"), "Select"=w814, "State(s) if False (\"\")"="Init: Elapsed Timer (TMS)" ("State(s) if False (\"\")")) -> ("States Out"=w818:string)  [unwired: 12 in]
        n314 = call <vilib>:"Add State(s) to Queue__jki_lib_state_machine.vi"("State(s) in Front (\"\")"=w818, "State(s) in (\"\")"=w837) -> ("States Out"=w836:string)  [unwired: 13 in]
      }
      frame "Init: Elapsed Timer (TMS)" {
        # "check if timer elased - if TRUE end test if FALSE read again."
        # "Template Separator\n(You can make a copy of, or modify, this frame)"
        # "Check to see if the timer has elpased."
        n315 = call "Timer.vi"("error in (no error)"=w845, "Target Time"=10.0, "Enum"=T4."Get Time") -> ("error out"=w844:errorcluster, "Time Elapsed?"=w841:bool, "Elapsed Time"=→"Timeout (Read States) 3":dbl)  [unwired: 5 in, 1 out]
        n316 = call-poly <vilib>:"Select State(s)__jki_lib_state_machine.vi"("State(s) if True (\"\")"="Init: Start Timer (WfS)" ("State(s) if True (\"\")"), "Select"=w841, "State(s) if False (\"\")"="Init: Read TMS State" ("State(s) if False (\"\")")) -> ("States Out"=w840:string)  [unwired: 12 in]
        n317 = call <vilib>:"Add State(s) to Queue__jki_lib_state_machine.vi"("State(s) in Front (\"\")"=w840, "State(s) in (\"\")"=w849) -> ("States Out"=w848:string)  [unwired: 13 in]
      }
      frame "Init: Start Timer (WfS)" {
        # "Start 10 second timer"
        # "Template Separator\n(You can make a copy of, or modify, this frame)"
        n318 = call "Timer.vi"("error in (no error)"=w856, "Enum"=T4."Start Timer") -> ("error out"=w855:errorcluster)  [unwired: 6 in, 3 out]
        n319 = property on="Timeout (Read States) 4" class="Slide (strict)"(error in=w855, "Value"=0.0 ("Horizontal Pointer Slide"), "Scale.Maximum"=10.0 ("Target Time"), "Scale.Minimum"=0.0 ("Scale.Range:Minimum")) -> (error out=w851:errorcluster)  [unwired: 1 in, 1 out]
        n320 = call <vilib>:"Add State(s) to Queue__jki_lib_state_machine.vi"("State(s) in Front (\"\")"="Init: Read Wait for Start State" ("State(s) in Front (\"\")"), "State(s) in (\"\")"=w860) -> ("States Out"=w859:string)  [unwired: 13 in]
      }
      frame "Init: Read Wait for Start State" {
        # "Read UDP if equal to F0 test complete if not check if timer has elapsed."
        # "#56 = didnt read before the timeout"
        # "Template Separator\n(You can make a copy of, or modify, this frame)"
        n321 = Unbundle By Name(w867) -> ("connection ID"=w880:refnum<k16>)
        n322 = UDP Read(connection ID=w880, timeout ms (25000)=1, 8:w862) -> (data out=w874:string, error out=w873:errorcluster, 3:w864:refnum<k16>)  [unwired: 1 in, 2 out]
        n323 = String Subset(string=w874, offset (0)=17 ("offset (0) 2"), length (rest)=1 ("length (rest) 2")) -> (substring=w876:string)
        n324 = String To Byte Array(string=w876) -> (unsigned byte array=w879:u8[])
        n325 = Number To Hexadecimal String(2:w879) -> (0:w878:string[])  [unwired: 1 in]
        n326 = Index Array(array=w878, index=0) -> (element=w868:string)
        n327 = Equal?(x=w868, y="15") -> (x = y?=w861:bool)
        "Wait for Start" <- w861
        n328 = call <vilib>:"Clear Errors.vi"("error in (no error)"=w873, "specific error code to clear (0: all)"=56) -> ("error out"=w863:errorcluster)  [unwired: 4 in, 1 out]
        n329 = Bundle By Name(cluster=w867, "connection ID"=w864, "Read Wait for Start"=w868) -> (w866:T5)
        n330 = call-poly <vilib>:"Select State(s)__jki_lib_state_machine.vi"("State(s) if True (\"\")"="Init: Start Command" ("State(s) if True (\"\")"), "Select"=w861, "State(s) if False (\"\")"="Init: Elapsed Timer (WfS)" ("State(s) if False (\"\")")) -> ("States Out"=w865:string)  [unwired: 12 in]
        n331 = call <vilib>:"Add State(s) to Queue__jki_lib_state_machine.vi"("State(s) in Front (\"\")"=w865, "State(s) in (\"\")"=w884) -> ("States Out"=w883:string)  [unwired: 13 in]
      }
      frame "Init: Elapsed Timer (WfS)" {
        # "check if timer elased - if TRUE end test if FALSE read again."
        # "Template Separator\n(You can make a copy of, or modify, this frame)"
        # "Check to see if the timer has elpased."
        n332 = call "Timer.vi"("error in (no error)"=w892, "Target Time"=10.0, "Enum"=T4."Get Time") -> ("error out"=w891:errorcluster, "Time Elapsed?"=w888:bool, "Elapsed Time"=→"Timeout (Read States) 4":dbl)  [unwired: 5 in, 1 out]
        n333 = call-poly <vilib>:"Select State(s)__jki_lib_state_machine.vi"("State(s) if True (\"\")"="Init: Start Command" ("State(s) if True (\"\")"), "Select"=w888, "State(s) if False (\"\")"="Init: Read Wait for Start State" ("State(s) if False (\"\")")) -> ("States Out"=w887:string)  [unwired: 12 in]
        n334 = call <vilib>:"Add State(s) to Queue__jki_lib_state_machine.vi"("State(s) in Front (\"\")"=w887, "State(s) in (\"\")"=w896) -> ("States Out"=w895:string)  [unwired: 13 in]
      }
      frame "Init: Start Command" {
        # "None"
        # "RIB Box IP"
        # "Data"
        # "Length"
        # "ID"
        # "Target"
        # "Type"
        # "Pkt ID"
        # "SET"
        # "Template Separator\n(You can make a copy of, or modify, this frame)"
        n335 = Unbundle By Name(w915) -> ("connection ID"=w903:refnum<k16>)
        n336 = Build Array(u8 91 ("element"), u8 1 ("element"), u8 9 ("element"), u8 110 ("element"), u8 0 ("element")) -> (w913:u8[])
        n337 = Byte Array To String(unsigned byte array=w913) -> (string=w914:string)
        n338 = String To IP(1:"192.168.201.21" ("name")) -> (0:w906:u32)
        n339 = UDP Write(address=w906, port or service name=u16 54321, connection ID=w903, data in=w914, 8:w904, 9:1000 ("timeout ms (25000)")) -> (error out=w899:errorcluster, 3:w902:refnum<k16>)
        n340 = Bundle By Name(cluster=w915, "connection ID"=w902) -> (w916:T5)
        n341 = call <userlib>:"Wait (ms)__ogtk.vi"("error in (no error)"=w899, "milliseconds to wait"=u32 1000) -> ("error out"=w898:errorcluster)  [unwired: 8 in, 1 out]
        n342 = call <vilib>:"Add State(s) to Queue__jki_lib_state_machine.vi"("State(s) in Front (\"\")"="Init: Read Normal Operation" ("State(s) in Front (\"\")"), "State(s) in (\"\")"=w918) -> ("States Out"=w917:string)  [unwired: 13 in]
      }
      frame "Init: Read Normal Operation" {
        # "Read UDP if equal to F0 test complete if not check if timer has elapsed."
        # "#56 = didnt read before the timeout"
        # "Template Separator\n(You can make a copy of, or modify, this frame)"
        n343 = Unbundle By Name(w927) -> ("connection ID"=w936:refnum<k16>)
        n344 = UDP Read(connection ID=w936, timeout ms (25000)=10, 8:w924) -> (data out=w930:string, error out=w929:errorcluster, 3:w925:refnum<k16>)  [unwired: 1 in, 2 out]
        n345 = String Subset(string=w930, offset (0)=17 ("offset (0) 2"), length (rest)=1 ("length (rest) 2")) -> (substring=w932:string)
        n346 = String To Byte Array(string=w932) -> (unsigned byte array=w935:u8[])
        n347 = Number To Hexadecimal String(2:w935) -> (0:w934:string[])  [unwired: 1 in]
        n348 = Index Array(array=w934, index=0) -> (element=w921:string)
        n349 = call <vilib>:"Clear Errors.vi"("error in (no error)"=w929, "specific error code to clear (0: all)"=56) -> ("error out"=w922:errorcluster)  [unwired: 4 in, 1 out]
        n350 = Equal?(x=w921, y="19") -> (x = y?=→"Normal Operation":bool)
        n351 = Bundle By Name(cluster=w927, "connection ID"=w925, "Read Normal Operation"=w921) -> (w926:T5)
        n352 = call <vilib>:"Add State(s) to Queue__jki_lib_state_machine.vi"("State(s) in Front (\"\")"="Macro: Limits" ("State(s) in Front (\"\")"), "State(s) in (\"\")"=w940) -> ("States Out"=w939:string)  [unwired: 13 in]
      }
    }
    n353 = Wait (ms)(milliseconds to wait=u32 2) -> ()  [unwired: 1 out]
  }
  "error out" <- w1
